vi "TLB Native Dynamic Events ver 0.14a.vi"() -> ()   [LabVIEW 2018]
uses:
  Labview Training Phase 2/Enum Controls/States for Action Engine.ctl
  TLB Type Definitions/State Type Definitions, for 0.26d versions and later.ctl
  TLB Type Definitions/Intruction Type Definitions.ctl
  TLB Type Definitions/Encoder cluster.ctl
  TLB Type Definitions/PING CLUSTER.ctl
  <vilib>/Studica/Studica Toolkit/NavX/NavX.lvlib
  <vilib>/Studica/Studica Toolkit/Background/DIO Channel.ctl
  Underlying VI's/NavX VI/navX type def.ctl
  <vilib>/myRIO/Instrument Drivers/Utilities/Utilities.lvlib
  <vilib>/Studica/Studica Toolkit/Background/I2C Channel.ctl
  TLB Type Definitions/Vision cluster.ctl
  <vilib>/NI_Real-Time Target Support.lvlib
  TLB Type Definitions/Stepper cluster.ctl
  Experimental VI's/Archived VI's/MOTOR CONTROL NO PID Type Def.ctl
  Underlying VI's/I2C Master VI/I2C MASTER Type Def.ctl
  Underlying VI's/I2C Master VI/I2C_MASTER_WRITE_NEW Type Def.ctl
  <vilib>/userdefined/High Color/IMAQdx.ctl
  Underlying VI's/I2C Master VI/Arduino_Interfacing.ctl
  TLB Type Definitions/Yaw Cluster.ctl
  Experimental VI's/Archived VI's/MOTOR CONTROL NO PID AE DATA ENTRY MODE Type def.ctl
  Experimental VI's/Archived VI's/MOTOR CONTROL NO PID AE DIRECTIONS type def.ctl
  Underlying VI's/Elasped Timer/Control.ctl
  TLB Type Definitions/Time cluster.ctl
  TLB Type Definitions/Y Stepper cluster.ctl
  Underlying VI's/Modified webcam FGV/Webcam AE.ctl
  <vilib>/Utility/RT CPU Load.ctl
panel:
  out "Cluster":T1
  out "Object Center Coordinates":cluster{"x":sgl, "y":sgl}
  out "Object detection cluster":T2
  out "Time up flag":bool
  out "Speed & distance":T3
  out "Task selection":u8
  in  "Object recognition mode":enum16{"Ball", "Soap", "Gel", "Pipe", "None"}(ring)
  out "NavX Readings":T4
  out "Arduino Data":T5
  out "CPU loads":T6[](array[typedef]) {"ISR (%)" format="%#.2f"; "Idle (%)" format="%#.2f"; "Background (%)" format="%#.2f"; "Normal (%)" format="%#.2f"; "Above Normal (%)" format="%#.2f"; "High (%)" format="%#.2g"; "Timed Structures (%)" format="%#.2g"; "Time Critical (%)" format="%#.2g"; "Total (%)" format="%#.2g"}
  out "Obstacle detected?":bool
  out "TASK ENABLE":bool
  out "Rising Edge":bool
  in  "Green LED":bool
  out "Obstacle detected":bool
  out "I2C Error":errorcluster
  out "State Logic":T7=enum."Startup"
  out "elements":T8[](array[typedef])
  in  "STOP TASK":bool
  in  "OK Button":bool
  in  "STOP":bool
  out "error out":errorcluster
  out "Action Queue Items":i32
  out "State Logic Queue Items":i32
  out "Action Queues items":string[](array[string])=["Hardware reset", "Software reset", ""]
  out "Action State":string
  # "VISION"
  # "System Health Status Update"
  # "TLB FRAMEWORK STATUS"
  # "Test Programme written by Calvin Loke    Dated: 28 Aug 2019\nTest Programme revised by Dr Alex See   Dated 30 Aug 2019\n\nRevision date: 20/03/2020\nProgramme version:   TLB Native Dynamic Events ver 0.14a"
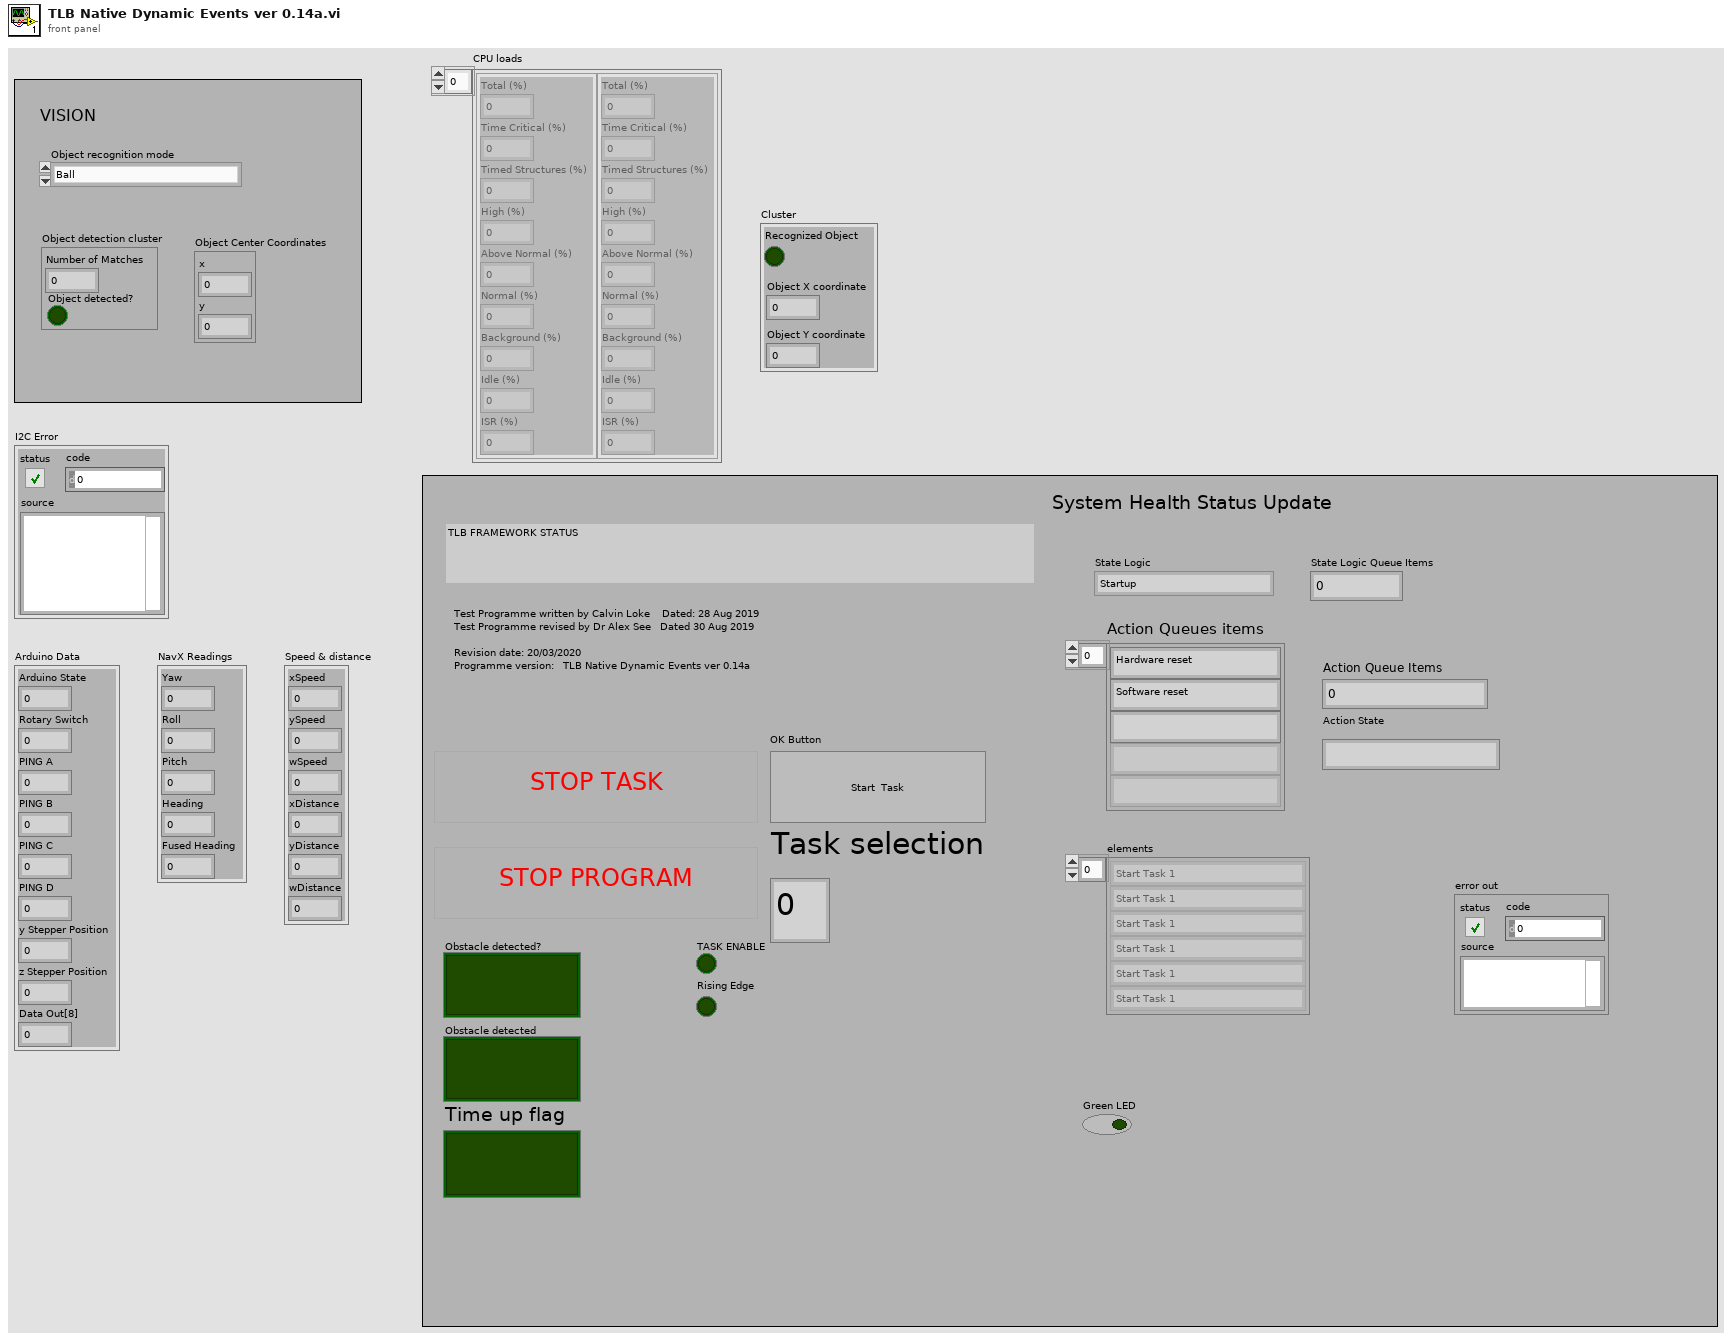
[diagram p1: front panel]
types:
  T1 = typedef "Vision cluster.ctl" = cluster{"Recognized Object":bool, "Object X coordinate":dbl, "Object Y coordinate":dbl}
  T2 = cluster{"Number of Matches":i32, "Object detected?":bool}
  T3 = cluster{"xSpeed":dbl, "ySpeed":dbl, "wSpeed":dbl, "xDistance":dbl, "yDistance":dbl, "wDistance":dbl}
  T4 = cluster{"Yaw":dbl, "Roll":dbl, "Pitch":dbl, "Heading":dbl, "Fused Heading":dbl}
  T5 = cluster{"Arduino State":u8, "Rotary Switch":u8, "PING A":u8, "PING B":u8, "PING C":u8, "PING D":u8, "y Stepper Position":u8, "z Stepper Position":u8, "Data Out[8]":u8}
  T6 = typedef "NI_Real-Time Target Support.lvlib/RT CPU Load.ctl" = cluster{"Total (%)":dbl, "Time Critical (%)":dbl, "Timed Structures (%)":dbl, "High (%)":dbl, "Above Normal (%)":dbl, "Normal (%)":dbl, "Background (%)":dbl, "Idle (%)":dbl, "ISR (%)":dbl}
  T7 = typedef "State Type Definitions.ctl" = enum16{"None", "Startup", "Move to Angle", "True Stop", "Idle", "Shutdown", "Task 1A", "Task 1B", "Task 2:Raise Arm", "Task 2:Sensor Mode", "Task 2:Reverse Mode", "Task 3", "Task 4_A", "Task 4_B", "Task 4_C", "Task 4_D", "Task 5A", "Task 5B", "Task 5C", "Task 5D", "Task 5E: POSITION ARM", "Task 5F: ARM GRAB HEIGHT", "Task 5G: CLOSE CLAW", "Task 5H: RAISE ARM", "Task 6_A", "Task 6_B", "Task 7", "Task 8A: RAISE ARM", "Task 8B: MOVE TO BOX", "Task 8C: CAM BURST", "Task 8D: PROCESS IMAGE", "Task 8E: ROBOT ADJUST", "Task 8F: CAM BURST 2", "Task 8G: PROCESS IMAGE 2", "Task 8H: ARM ADJUST", "Task 8I: ARM GRAB HEIGHT", "Task 8J: CLOSE CLAW", "Task 8K: RAISE MY SWORD", "Task 9A: Raise Arm", "Task 9B: Rotate to Angle", "Task 9C: Detect Box", "Task 9D: MOVE FORWARD", "Task 9E: MOVE LEFT", "Task 9F: SCAN IMAGE", "Task 9G: PROCESS COLOUR", "Task 9H: MOVE RIGHT", "Task 9I: SCAN IMAGE", "Task 9J: PROCESS COLOUR", "Task 9K: ROTATE 90 CW", "Task 9L: MOVE FORWARD", "Task 9M: MOVE RIGHT", "Task 9N: SCAN IMAGE", "Task 9O: PROCESS COLOUR", "Task 9P: MOVE RIGHT", "Task 9Q: SCAN IMAGE", "Task 9R: PROCESS COLOUR", "Task A1: Raise Arm", "Task A2: Rotate to Angle", "Task A3: Move Forward", "Task A4: Rotate CW 90"}
  T8 = typedef "Intruction Type Definitions.ctl" = enum16{"None", "Start Task 1", "Start Task 2", "Start Task 3", "Start Task 4", "Start Task 5", "Start Task 6", "Start Task 7", "Start Task 8 - BALL", "Start Task 8 - Gel", "Start Task 8 - Pipe", "Start Task 8 - Soap", "Start Task 9", "Start Task A", "Start Task B", "Exit"}
  T9 = typedef "Y Stepper cluster.ctl" = cluster{"yStepper desired":u8}
  T10 = typedef "Time cluster.ctl" = cluster{"Time up flag":bool, "SET TIME TO CHECK":dbl}
  T11 = typedef "Yaw Cluster.ctl" = cluster{"Yaw":dbl, "Compass":dbl}
  T12 = typedef "Stepper cluster.ctl" = cluster{"y Stepper Position":u8, "z Stepper Position":u8}
  T13 = typedef "DIO Channel.ctl" = enum16{"Not Connected", "A/DIO1", "A/DIO2", "A/DIO3", "A/DIO4", "A/DIO5", "A/DIO6", "A/DIO7", "A/DIO13", "B/DIO1", "B/DIO2", "B/DIO3", "B/DIO4", "B/DIO5", "B/DIO6", "B/DIO7", "B/DIO13", "C/DIO0", "C/DIO1", "C/DIO2", "C/DIO3", "C/DIO4", "C/DIO5", "C/DIO6", "C/DIO7"}
  T14 = typedef "PING CLUSTER.ctl" = cluster{"PING_A":u8, "PING_B":u8, "PING_C":u8, "PING_D":u8}
  T15 = typedef "Encoder cluster.ctl" = cluster{"xDistance":dbl, "yDistance":dbl, "wDistance":dbl}
  T16 = cluster{"DIO Channel":T13, "FPGA VI Reference Out":refnum<k20>}
  T17 = typedef "MOTOR CONTROL NO PID AE DATA ENTRY MODE Type def.ctl" = enum16{"Initialize", "Reset Encoders", "Write to motors", "Read from Encoders"}
  T18 = typedef "navX type def.ctl" = enum16{"Get i2C reference", "Read Values", "Zero Yaw"}
  T19 = typedef "Arduino_Interfacing.ctl" = enum16{"Initialize", "Write to Arduino", "Read From Arduino"}
  T20 = typedef "I2C Channel.ctl" = enum16{"Not Connected", "A", "B"}
  T21 = typedef "States for Action Engine.ctl" = enum16{"Initialize", "Write", "Read"}
  T22 = cluster{"I2C Ref Out":cluster{"I2C Channel":T20, "FPGA VI Reference Out":refnum<k20>}, "Connected":bool, "Slave Address (7-bit)":u8, "Registry":u8[]}
  T23 = typedef "IMAQ Image.ctl" = refnum<image>
  T24 = typedef "State Type Definitions.ctl" = enum16{"None", "Startup", "Move to Angle", "True Stop", "Idle", "Shutdown", "Task 1", "Task 2", "Task 3", "Task 4_A", "Task 4_B", "Task 4_C", "Task 4_D", "Task 5_A", "Task 5 _B", "Task 5_C", "Task 5_D", "Task 5_D_Error", "Task 5D_Error_Right", "Task 5D_Error_Left", "Task 5_E", "Task 5_F", "Task 5F_Error", "Task 5G", "Task 5H", "Task 6_A", "Task 6_B", "Task 7", "Task 8", "Task 9", "Task A", "Task B"}
  T25 = typedef "State Type Definitions.ctl" = enum16{"None", "Startup", "Move to Angle", "True Stop", "Idle", "Shutdown", "Task 1", "Task 2", "Task 3", "Task 4_A", "Task 4_B", "Task 4_C", "Task 5_A", "Task 5 _B", "Task 5_C", "Task 5_C_Error", "Task 5_D", "Task 6_A", "Task 6_B", "Task 7", "Task 8", "Task 9", "Task A", "Task B"}
  T26 = typedef "MOTOR CONTROL NO PID AE DIRECTIONS type def.ctl" = enum16{"y-axis movement", "x-axis movement", "Rotate", "Stop"}
  T27 = typedef "Control.ctl" = enum16{"Start", "Pause", "Initialize"}
  T28 = typedef "I2C_MASTER_WRITE_NEW Type Def.ctl" = enum16{"Ultrasonic sensors", "Stepper origin", "zStepper 13.3k", "zStepper 13k", "zStepper 12k", "zStepper 11k", "zStepper 10k", "zStepper 9k", "zStepper 8k", "zStepper 7k", "zStepper 6k", "zStepper 5k", "zStepper 4k", "zStepper 3k", "zStepper 2k", "zStepper 1k", "zStepper 900", "zStepper 800", "zStepper 700", "zStepper 600", "zStepper 500", "zStepper 400", "zStepper 300", "zStepper 200", "zStepper 100", "zStepper 0", "yStepper control", "Open Claw", "Close Claw", "Soft Reset"}
  T29 = typedef "Webcam AE.ctl" = enum16{"Initialize Camera", "Open Camera", "Continuous Acquisition", "Close Camera", "Retrieve Image", "Dispose Camera Image Buffer"}
  T30 = typedef "IMAQdx.ctl" = refnum<k21>
  T31 = typedef "Webcam AE.ctl" = enum16{"Initialize Camera", "Open Camera", "Continuous Acquisition", "Close Camera", "Retrieve Image", "Dispose Image Buffers"}
  T32 = typedef "MOTOR CONTROL NO PID Type Def.ctl" = enum16{"Init", "Front Back", "Left Right", "Rotate", "Stop", "Latch"}
  T33 = typedef "I2C MASTER Type Def.ctl" = enum16{"Last State", "Mode 0", "Mode 1", "Mode 2", "Mode 3", "Mode 4", "Mode 5", "Mode 6", "Mode 7", "Mode 8", "Mode 9", "Mode 10"}
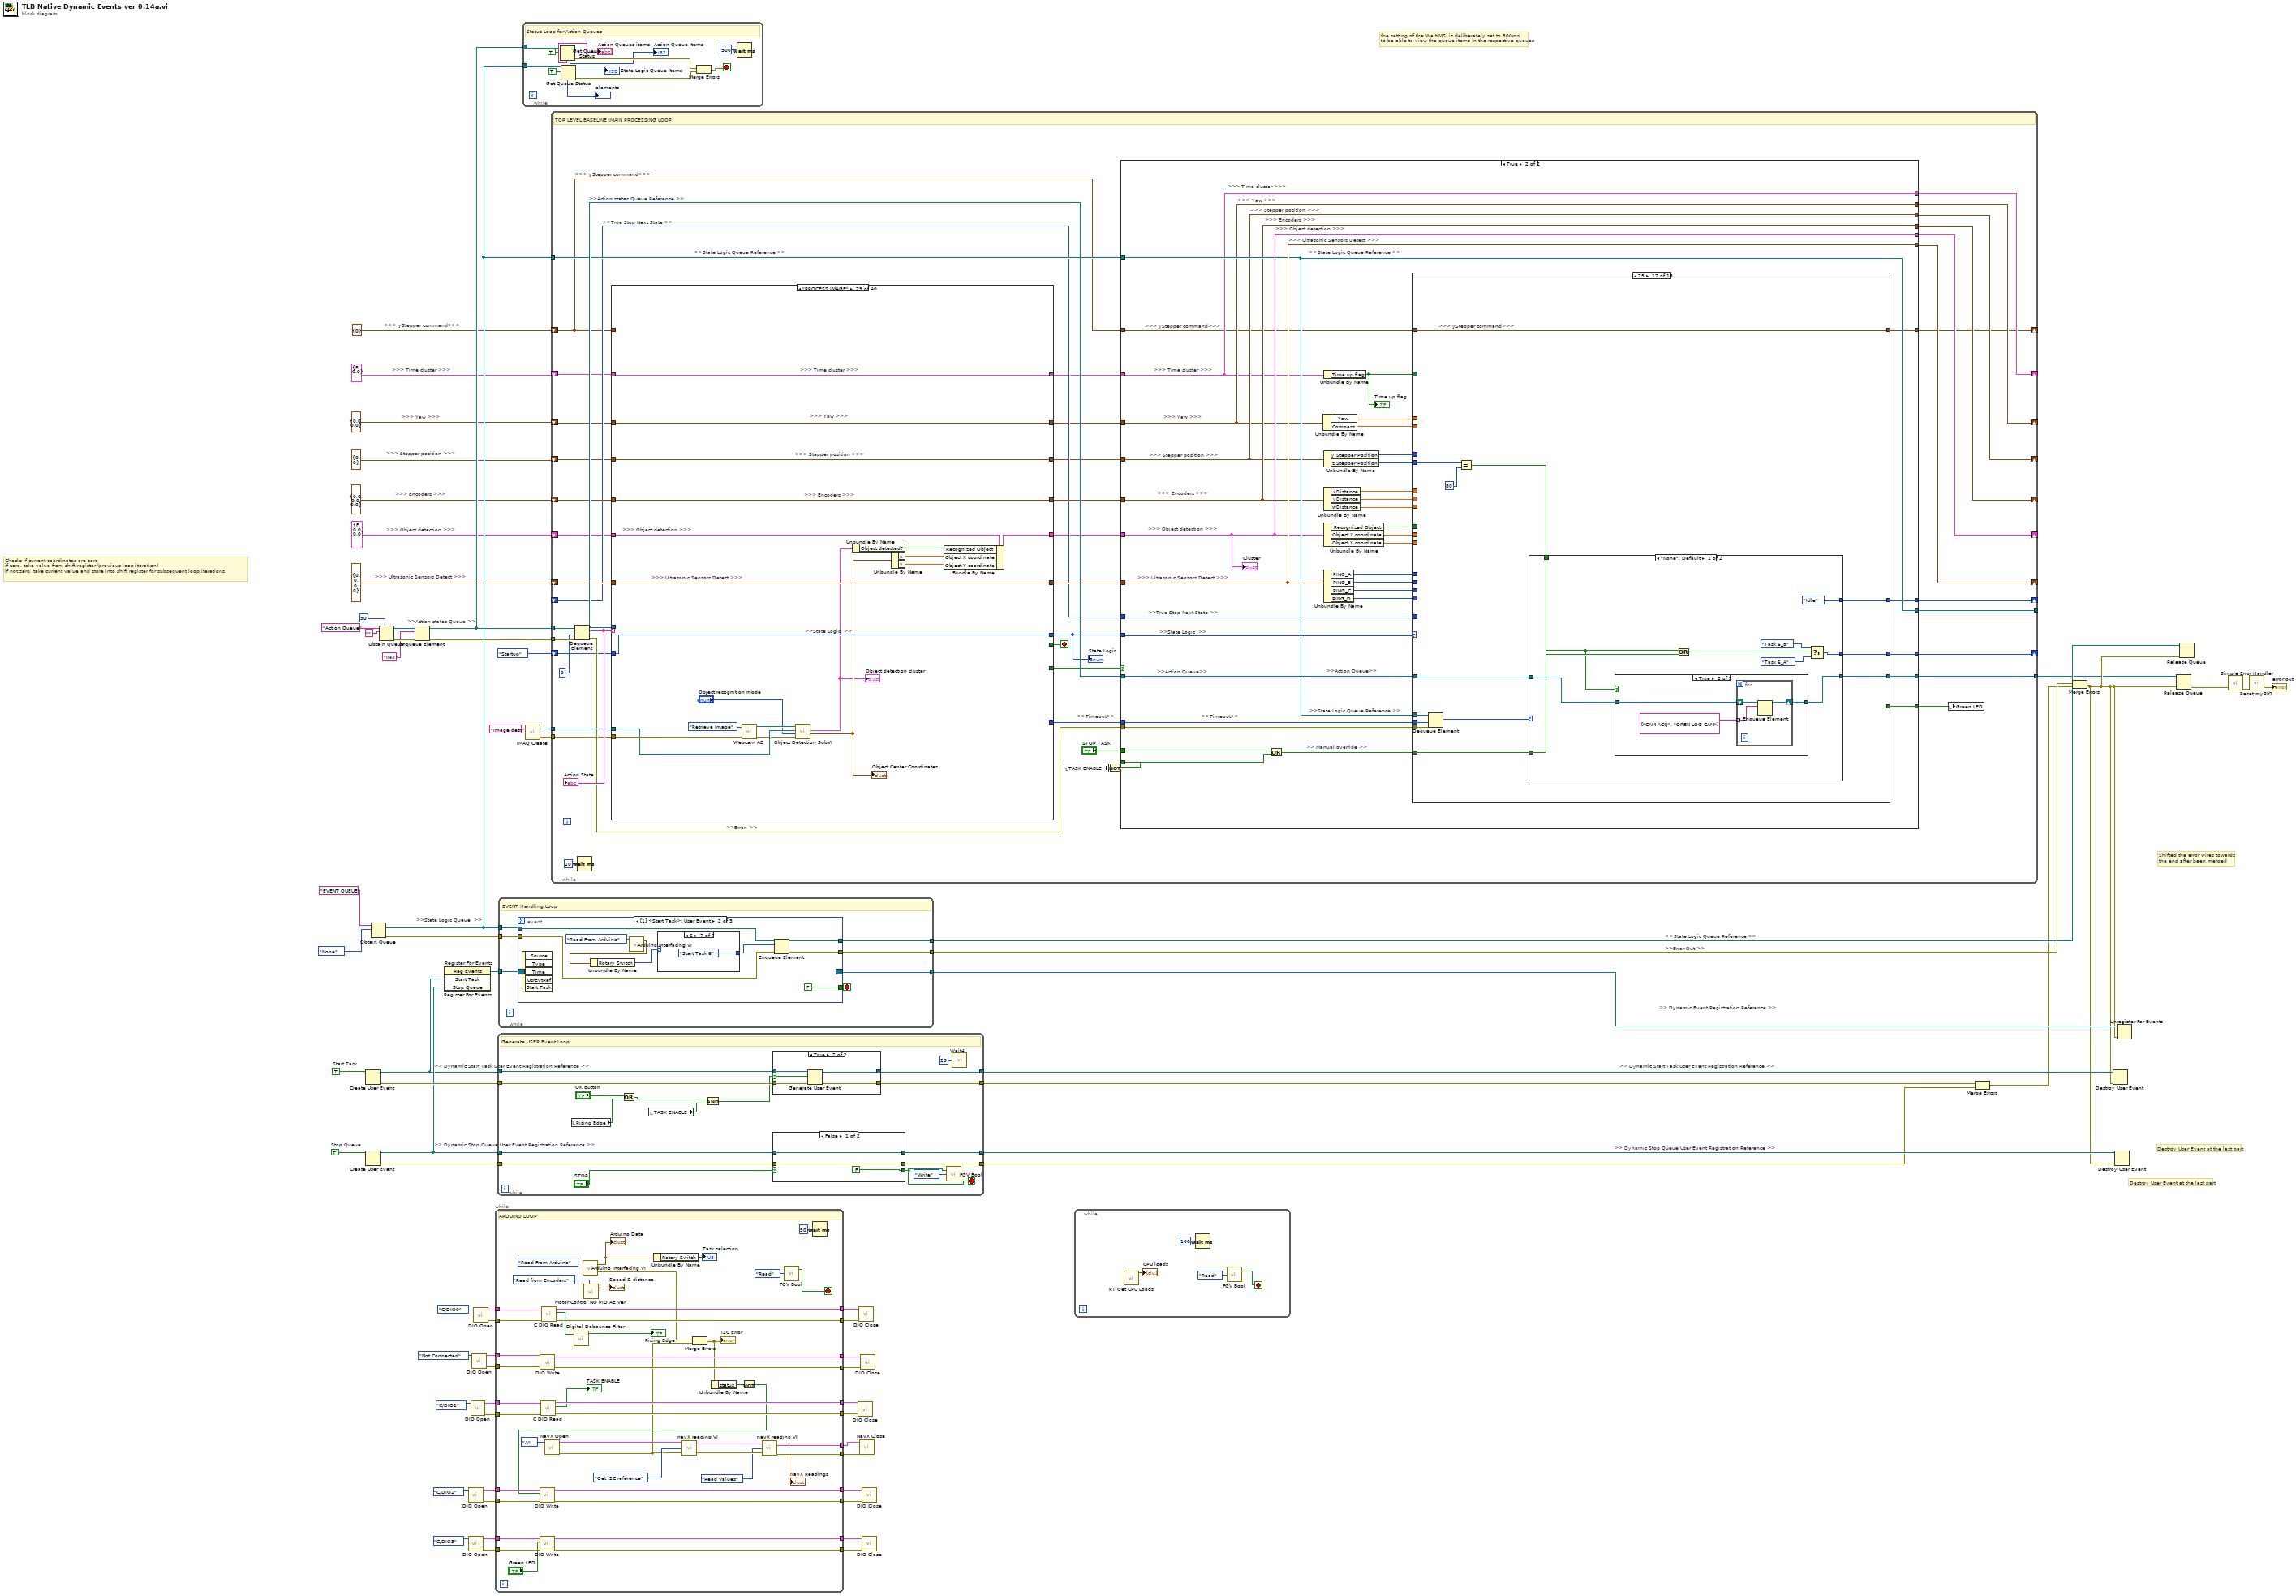
[diagram p0: block diagram]
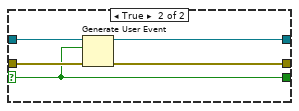
[diagram p2: hidden frame]
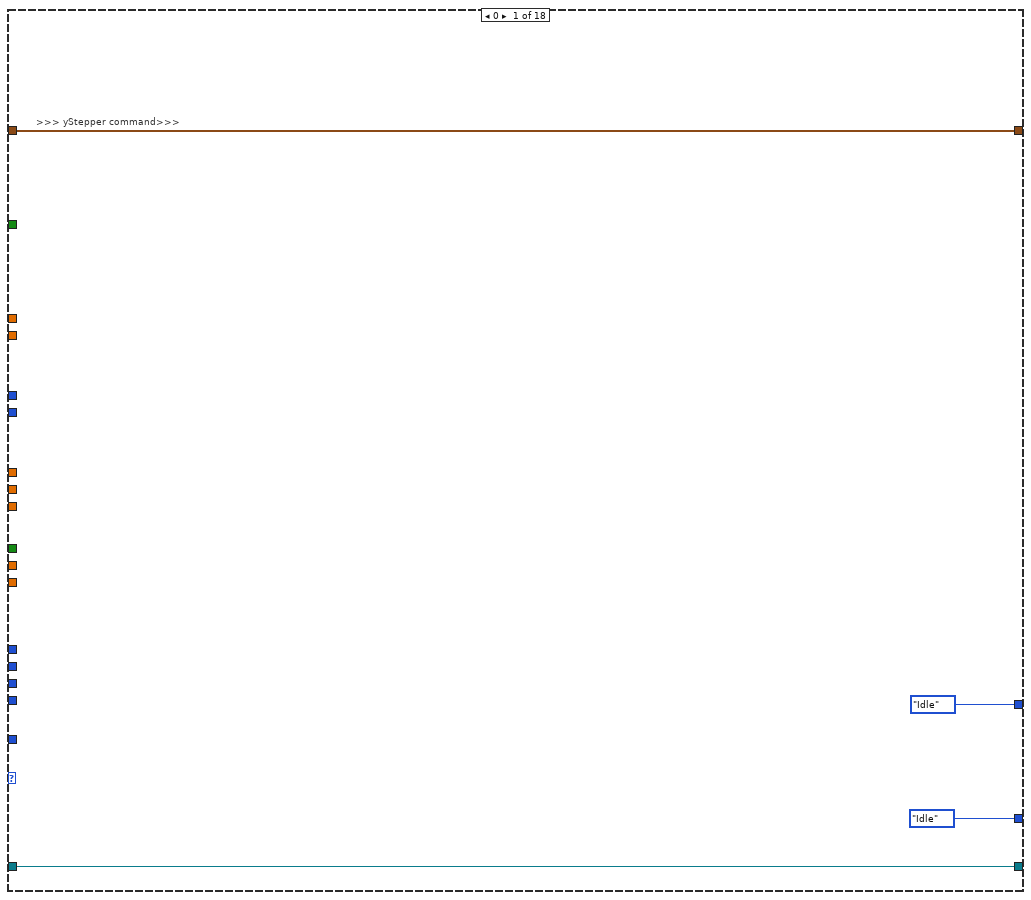
[diagram p5: hidden frame]
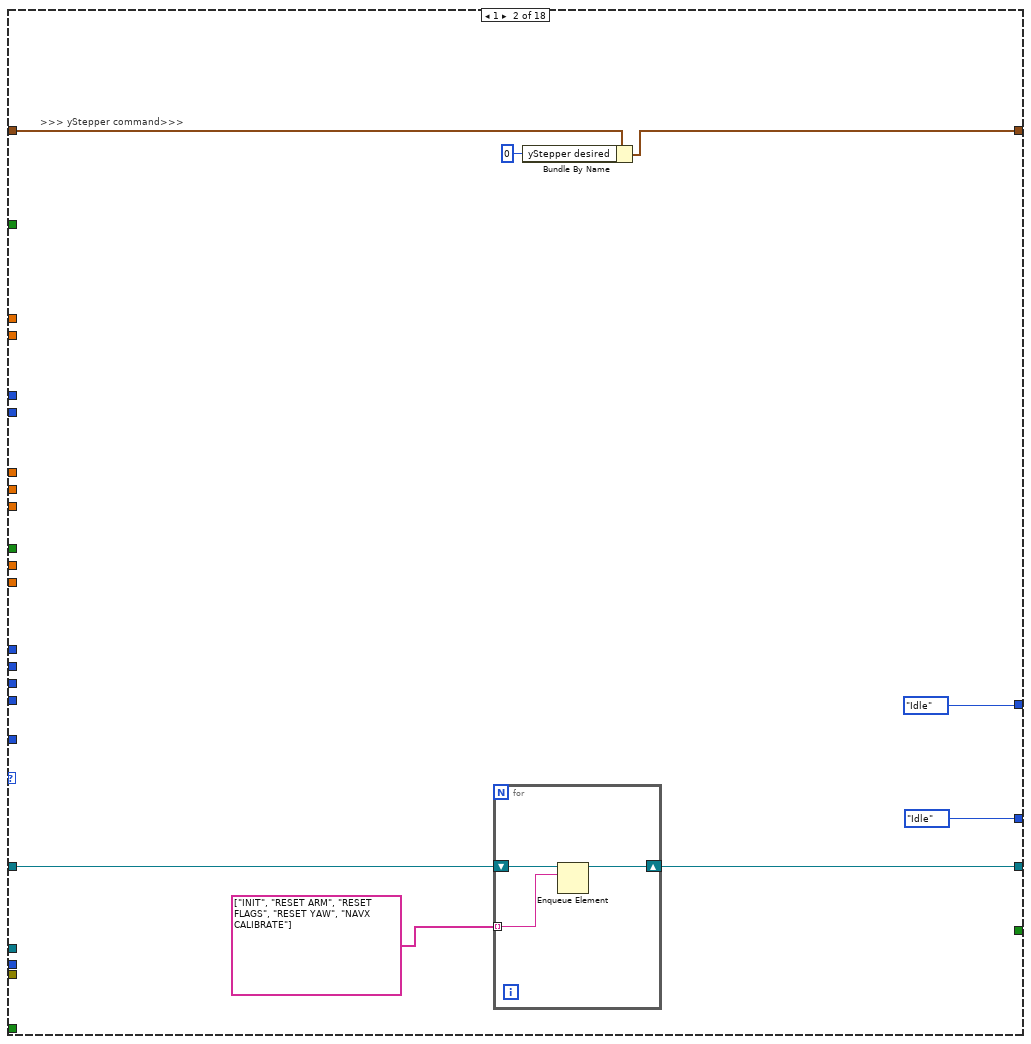
[diagram p6: hidden frame]
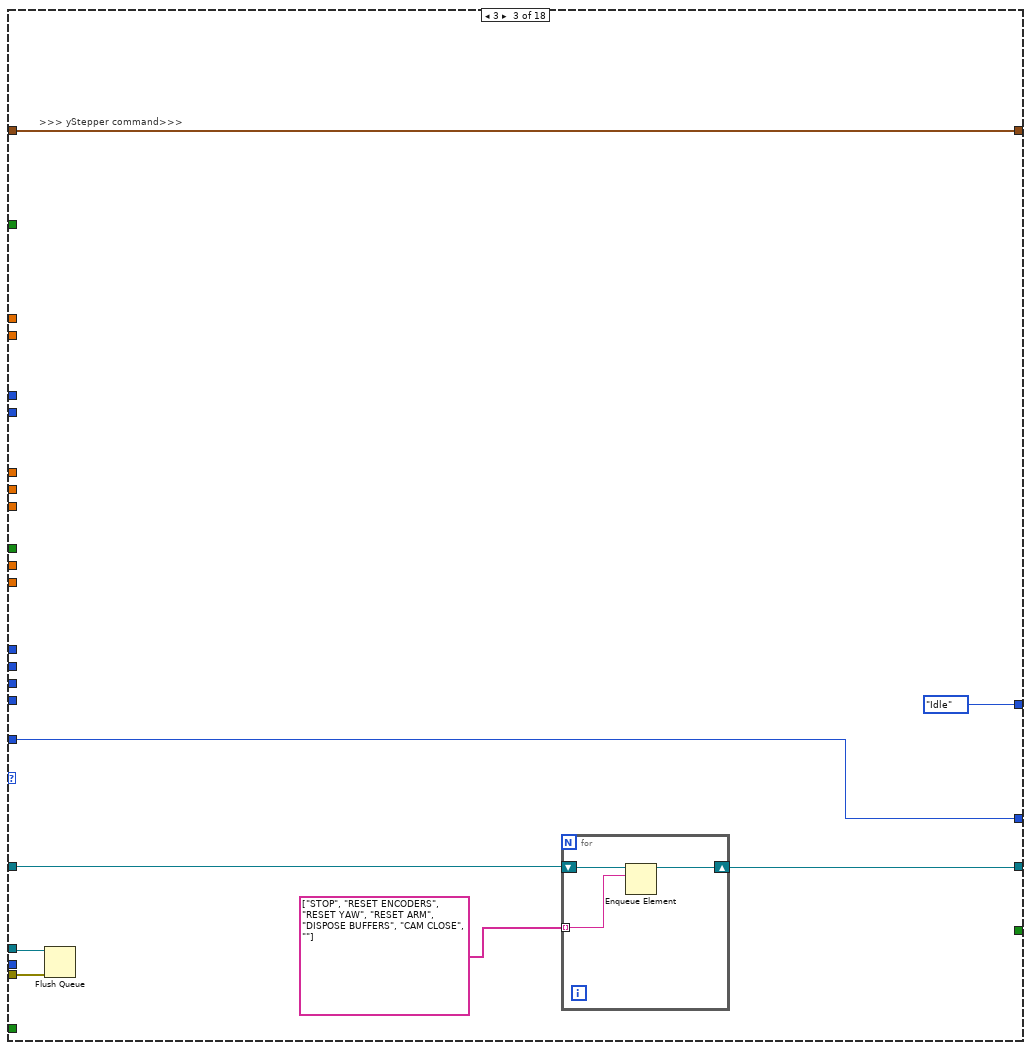
[diagram p7: hidden frame]
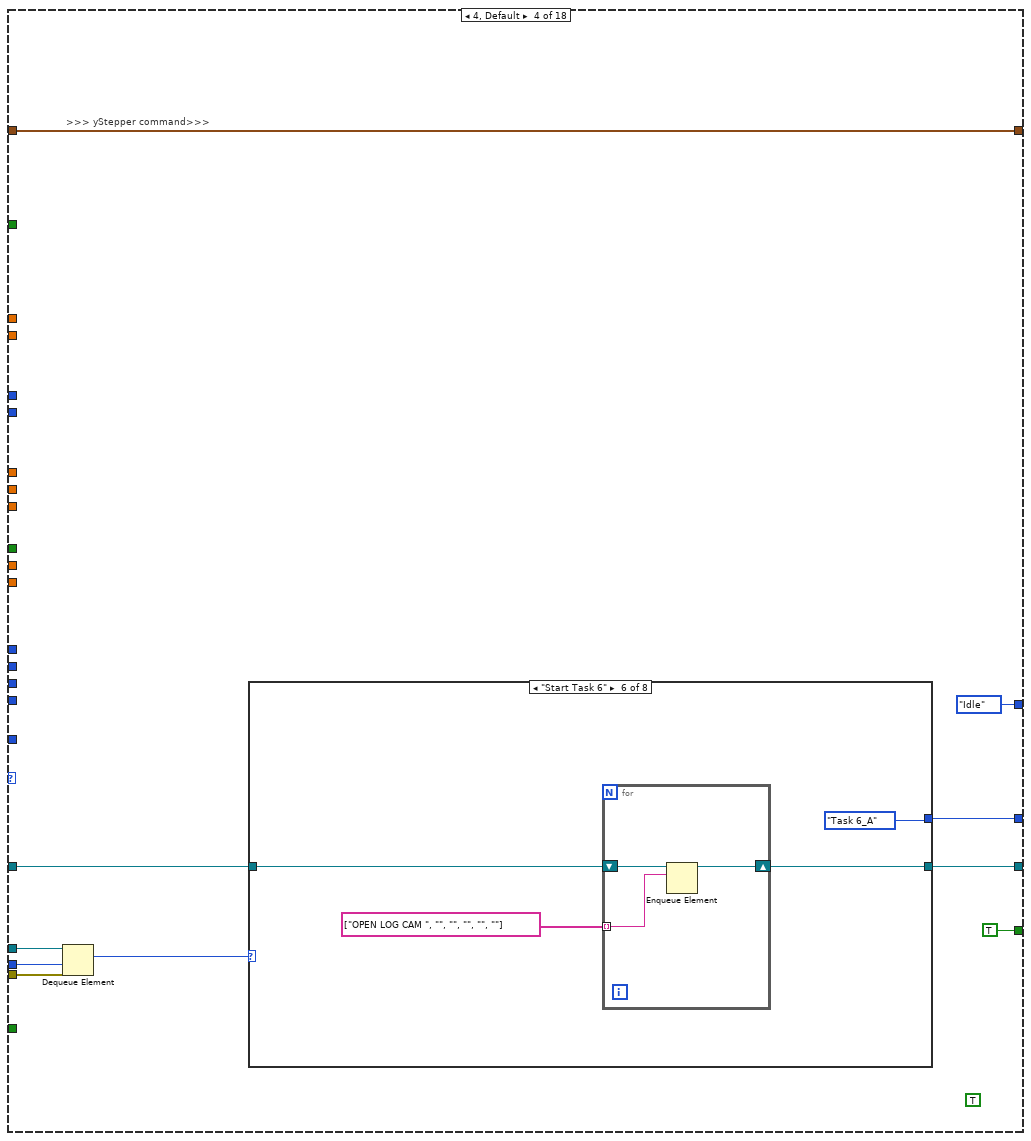
[diagram p8: hidden frame]
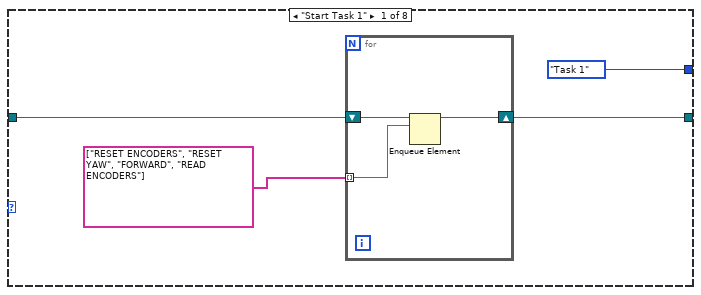
[diagram p9: hidden frame]
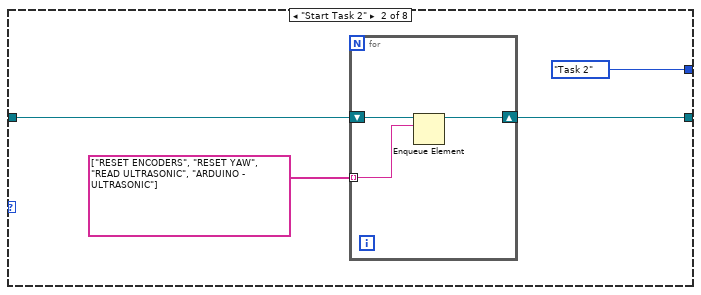
[diagram p10: hidden frame]
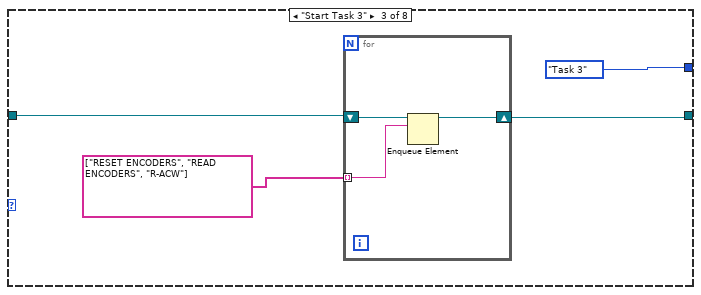
[diagram p11: hidden frame]
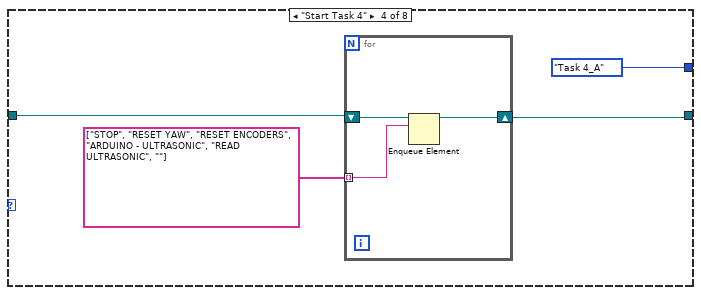
[diagram p12: hidden frame]
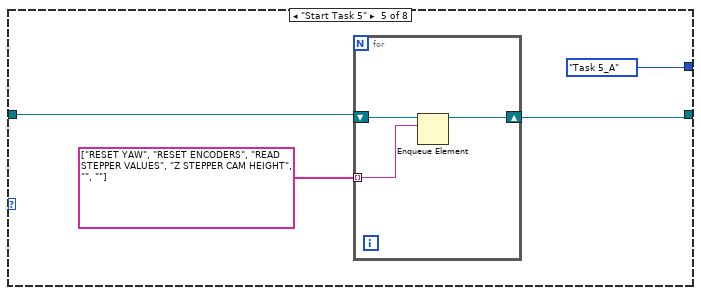
[diagram p13: hidden frame]
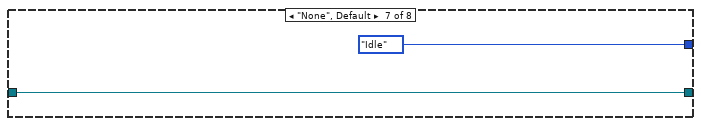
[diagram p14: hidden frame]
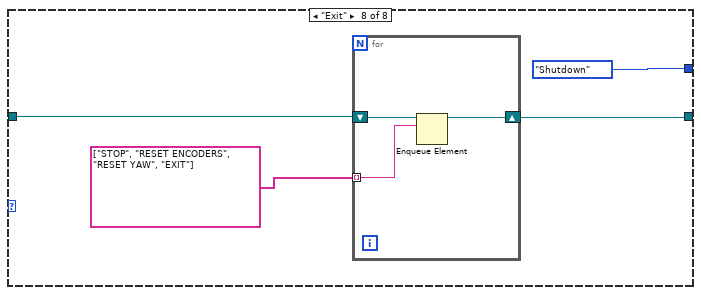
[diagram p15: hidden frame]
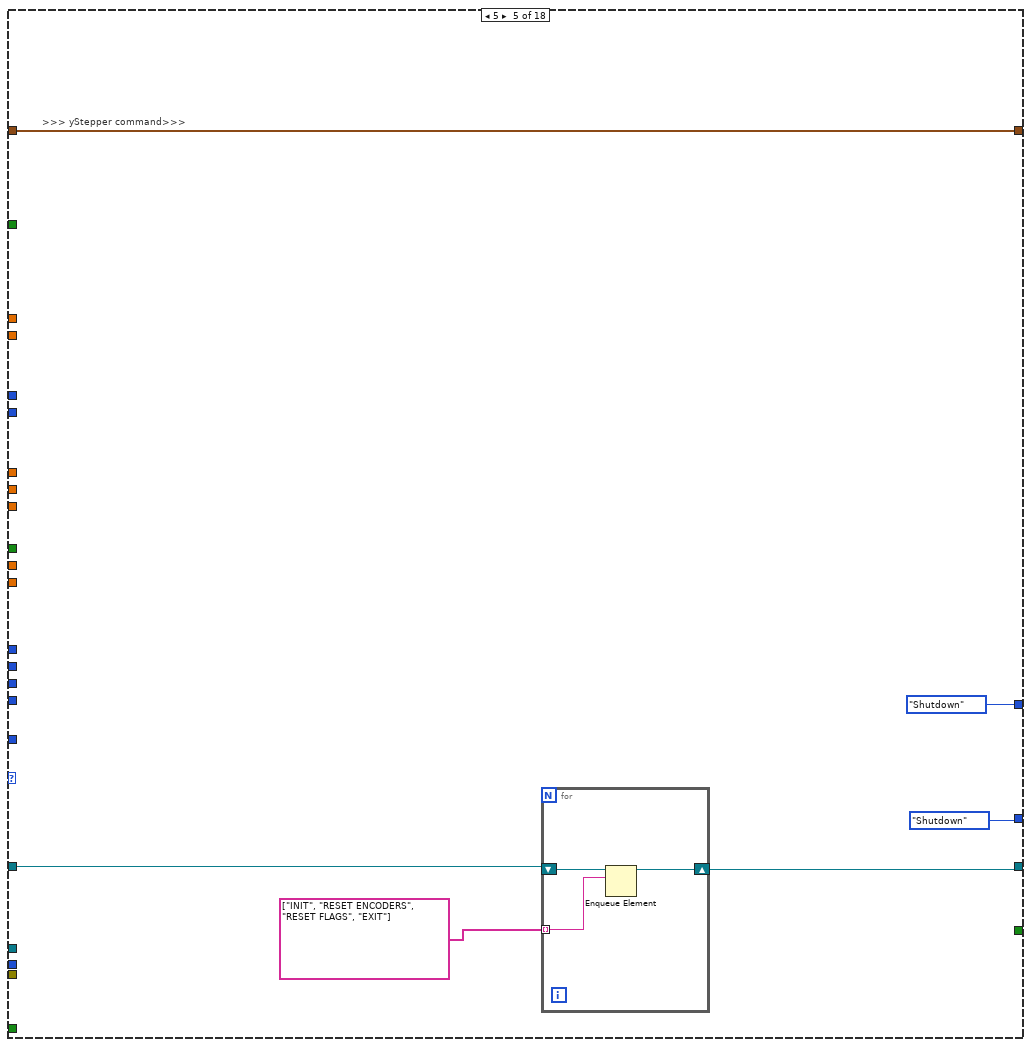
[diagram p16: hidden frame]
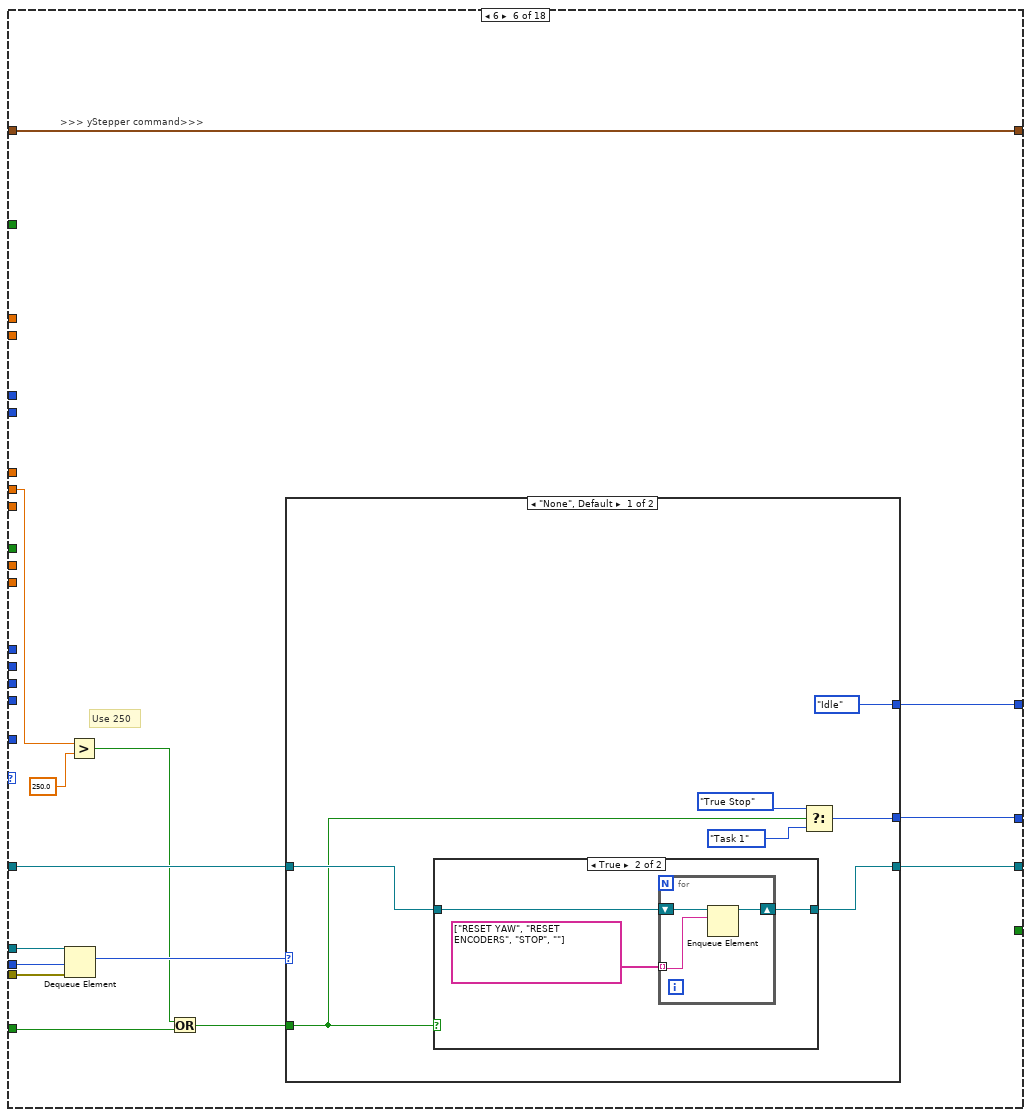
[diagram p17: hidden frame]
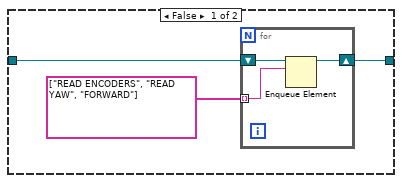
[diagram p18: hidden frame]
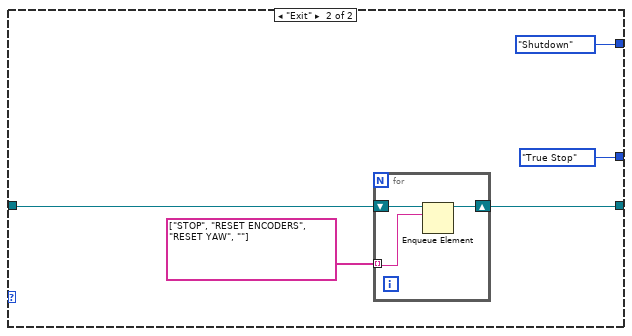
[diagram p19: hidden frame]
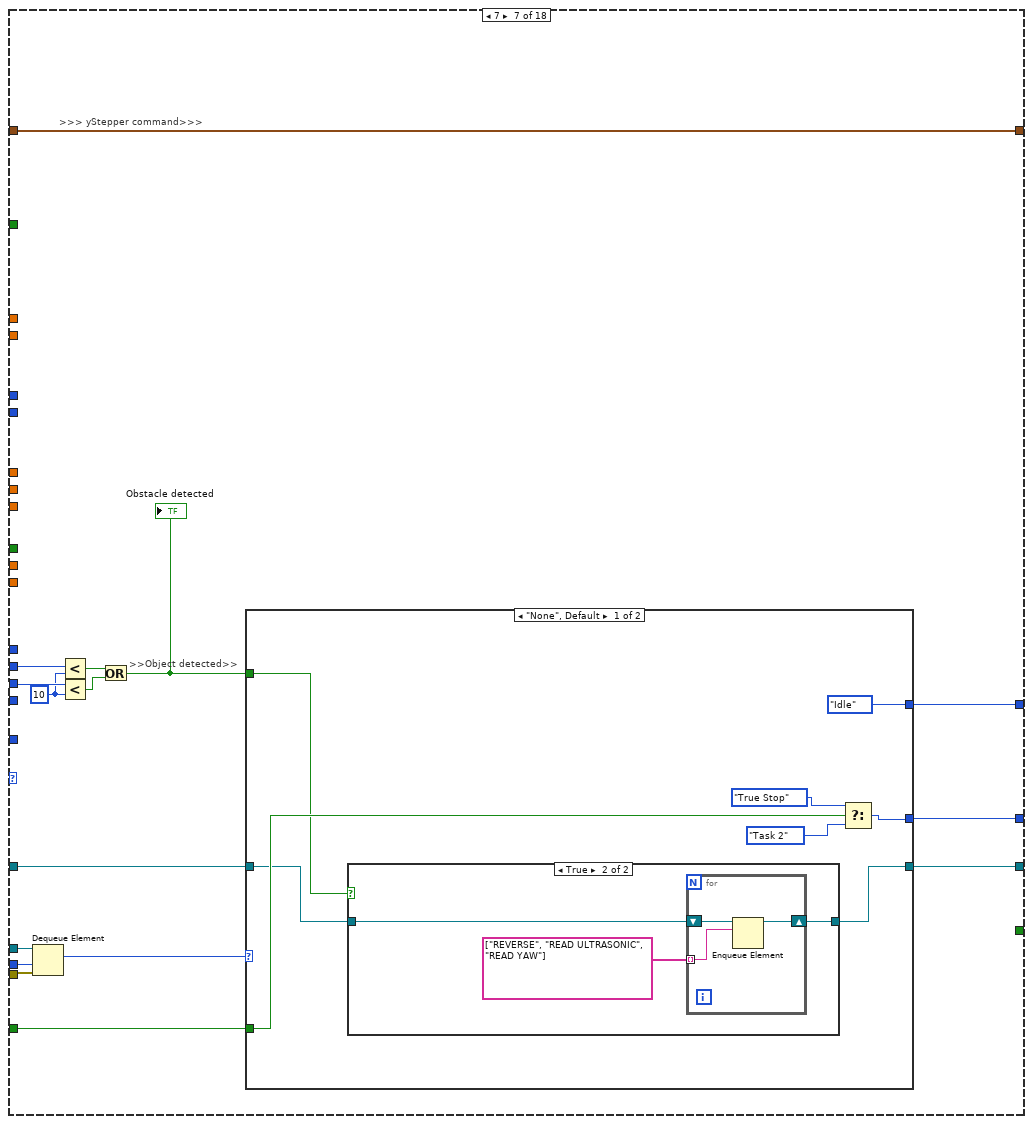
[diagram p20: hidden frame]
diagram:
  w70 = TRUE  # Stop Queue
  w69 = TRUE  # Start Task
  # "Checks if current coordinates are zero\nif zero, take value from shift register (previous loop iteration)\nif not zero, take current value and store into shift register for subsequent loop iterations"
  # ">>> yStepper command>>>"
  # ">>> Time cluster >>>"
  # ">>> Yaw >>>"
  # ">>> Stepper position >>>"
  # ">>> Encoders >>>"
  # ">>> Object detection >>>"
  # ">>> Ultrasonic Sensors Detect >>>"
  # "the setting of the Wait(MS) is deliberately set to 500ms\nto be able to view the queue items in the respective queues"
  # ">>Error Out >>"
  # ">> Dynamic Stop Queue User Event Registration Reference >>"
  # ">> Dynamic Start Task User Event Registration Reference >>"
  # ">> Dynamic Stop Queue User Event Registration Reference >>"
  # ">> Dynamic Start Task User Event Registration Reference >>"
  # ">> Dynamic Event Registration Reference >>"
  # ">>Action states Queue >>"
  # ">>State Logic Queue  >>"
  # ">>State Logic Queue Reference >>"
  # "Destroy User Event at the last part"
  # "Destroy User Event at the last part"
  # "Shifted the error wires towards\nthe end after been merged"
  n1 = Create User Event(user event datatype=w69) -> (user event=w61:refnum<user-event>, error out=w66:errorcluster)  [unwired: 1 in]
  n2 = Create User Event(user event datatype=w70) -> (user event=w62:refnum<user-event>, error out=w65:errorcluster)  [unwired: 1 in]
  n3 = Obtain Queue(name (unnamed)="EVENT QUEUE", element data type=Intruction_Type_Definitions."None" ("Enum")) -> (queue out=w47:refnum<queue>, error out=w53:errorcluster)  [unwired: 3 in, 1 out]
  n4 = Obtain Queue(max queue size (-1, unlimited)=50, name (unnamed)="Action Queue", element data type="") -> (queue out=w56:refnum<queue>, error out=w52:errorcluster)  [unwired: 2 in, 1 out]
  n5 = Enqueue Element(queue=w56, element="INIT", error in (no error)=w52) -> (queue out=w48:refnum<queue>, error out=w51:errorcluster)  [unwired: 1 in, 1 out]
  n6 = register-events "Register For Events"(w61, w62) -> (reference out=w60:refnum<event-registration>)  [unwired: 2 in, 1 out]
  n7 = call <vilib>:"DIO Open.vi"("DIO Channel"=DIO_Channel."C/DIO2") -> ("error out"=w14:errorcluster, "DIO Info Out"=w15:T16)  [unwired: 9 in]
  n8 = call <vilib>:"DIO Open.vi"("DIO Channel"=DIO_Channel."C/DIO3") -> ("error out"=w9:errorcluster, "DIO Info Out"=w10:T16)  [unwired: 9 in]
  n9 = call <vilib>:"DIO Open.vi"("DIO Channel"=DIO_Channel."C/DIO1") -> ("error out"=w25:errorcluster, "DIO Info Out"=w26:T16)  [unwired: 9 in]
  n10 = call <vilib>:"DIO Open.vi"("DIO Channel"=DIO_Channel."Not Connected") -> ("error out"=w30:errorcluster, "DIO Info Out"=w32:T16)  [unwired: 9 in]
  n11 = call <vilib>:"DIO Open.vi"("DIO Channel"=DIO_Channel."C/DIO0") -> ("error out"=w35:errorcluster, "DIO Info Out"=w38:T16)  [unwired: 9 in]
  n12 = while {
    tunnel: w38 -> [w113]
    tunnel: [w112] -> w36
    tunnel: w35 -> [w111]
    tunnel: [w110] -> w34
    tunnel: w32 -> [w107]
    tunnel: [w106] -> w31
    tunnel: w30 -> [w105]
    tunnel: [w104] -> w29
    tunnel: [w103] -> w27
    tunnel: w26 -> [w102]
    tunnel: w25 -> [w101]
    tunnel: [w100] -> w24
    tunnel: w15 -> [w94]
    tunnel: w14 -> [w93]
    tunnel: [w92] -> w13
    tunnel: [w91] -> w12
    tunnel: w10 -> [w90]
    tunnel: w9 -> [w89]
    tunnel: [w88] -> w8
    tunnel: [w87] -> w7
    tunnel: [w81] -> w4
    tunnel: [w80] -> w5
    stop <- w115 stop-if-true
    # "ARDUINO LOOP"
    n13 = call <vilib>:"DIO Write.vi"("error in (no error)"=w89, "Input"="Green LED", "DIO Info In"=w90) -> ("error out"=w87:errorcluster, "DIO Info Out"=w88:T16)  [unwired: 7 in]
    n14 = call <vilib>:"DIO Write.vi"("error in (no error)"=w105, "DIO Info In"=w107) -> ("error out"=w104:errorcluster, "DIO Info Out"=w106:T16)  [unwired: 8 in]
    n15 = call <vilib>:"C DIO Read.vi"("error in (no error)"=w101, "DIO Info In in"=w102) -> ("error out"=w100:errorcluster, "IN"=→"TASK ENABLE":bool, "DIO Info In out"=w103:T16)  [unwired: 7 in]
    n16 = call <vilib>:"C DIO Read.vi"("error in (no error)"=w111, "DIO Info In in"=w113) -> ("error out"=w110:errorcluster, "IN"=w109:bool, "DIO Info In out"=w112:T16)  [unwired: 7 in]
    n17 = call <vilib>:"NavX Open.vi"("I2C Channel"=I2C_Channel."A") -> ("error out"=w96:errorcluster, "NavX Info"=w98:T22)  [unwired: 9 in]
    n18 = call "Digital Debounce Filter.vi"("Boolean input"=w109) -> ("Rising Edge"=→"Rising Edge":bool)  [unwired: 1 in, 2 out]
    n19 = call "Arduino Interfacing VI.vi"("AE Mode"=Arduino_Interfacing."Read From Arduino") -> ("error out"=w84:errorcluster, "Arduino Data"=w77:T5)  [unwired: 3 in]
    "Arduino Data" <- w77
    n20 = call "Motor Control NO PID AE Ver.vi"("AE Mode"=MOTOR_CONTROL_NO_PID_AE_DATA_ENTRY_MODE_Type_def."Read from Encoders") -> ("Speed & distance"=→"Speed & distance":T3)  [unwired: 4 in, 1 out]
    n21 = Unbundle By Name(w77) -> ("Rotary Switch"=→"Task selection":u8)
    n22 = call "navX reading VI.vi"("NavX Info In"=w98, "Mode"=navX_type_def."Get i2C reference", "error in (no error)"=w96) -> ("NavX Info Out"=w83:T22, "Error Out"=w82:errorcluster)  [unwired: 2 out]
    n23 = Merge Errors(w84, w96) -> (w73:errorcluster)
    "I2C Error" <- w73
    n24 = Unbundle By Name(w73) -> ("status"=w72:bool)
    n25 = Not(x=w72) -> (.not. x?=w71:bool)
    n26 = call <vilib>:"DIO Write.vi"("error in (no error)"=w93, "Input"=w71, "DIO Info In"=w94) -> ("error out"=w91:errorcluster, "DIO Info Out"=w92:T16)  [unwired: 7 in]
    n27 = call "navX reading VI.vi"("NavX Info In"=w83, "Mode"=navX_type_def."Read Values", "error in (no error)"=w82) -> ("NavX Info Out"=w81:T22, "NavX Readings"=→"NavX Readings":T4, "Error Out"=w80:errorcluster)  [unwired: 1 out]
    n28 = call "FGV Bool.vi"("Init/Read/Write State"=States_for_Action_Engine."Read") -> ("Output node"=w115:bool)  [unwired: 2 in, 1 out]
    n29 = Wait (ms)(milliseconds to wait=u32 50) -> ()  [unwired: 1 out]
  }
  n30 = while {
    tunnel: w61 -> [w133]
    tunnel: w62 -> [w132]
    tunnel: [w131] -> w68
    tunnel: [w130] -> w67
    tunnel: w66 -> [w129]
    tunnel: [w128] -> w64
    tunnel: w65 -> [w127]
    tunnel: [w126] -> w63
    stop <- w124 stop-if-true
    # "Generate USER Event Loop"
    n31 = local read "Rising Edge"() -> (w120:bool)
    n32 = Or(x="OK Button", y=w120) -> (x .or. y?=w119:bool)
    n33 = local read "TASK ENABLE"() -> (w118:bool)
    n34 = And(x=w119, y=w118) -> (x .and. y?=w117:bool)
    n35 = case shown="True" w117 {
      selector: w117 -> [_ w144]
      tunnel: w133 -> [w143 w148]
      tunnel: [w143 w147] -> w130
      tunnel: w129 -> [w142 w146]
      tunnel: [w142 w145] -> w128
      frame False {
      }
      frame True {
        n36 = Generate User Event(user event=w148, event data cluster=w144, error in=w146) -> (user event out=w147:refnum<user-event>, error out=w145:errorcluster)  [unwired: 1 in]
      }
    }
    n37 = case shown="False" "STOP" {
      selector: "STOP" -> [_ w137]
      tunnel: w132 -> [w136 w141]
      tunnel: [w136 w140] -> w131
      tunnel: w127 -> [w135 w139]
      tunnel: [w135 w138] -> w126
      tunnel: [FALSE w137] -> w124
      frame False {
      }
      frame True {
        n38 = Generate User Event(user event=w141, event data cluster=w137, error in=w139) -> (user event out=w140:refnum<user-event>, error out=w138:errorcluster)  [unwired: 1 in]
      }
    }
    n39 = call "FGV Bool.vi"("Init/Read/Write State"=States_for_Action_Engine."Write", "Input Node"=w124) -> ()  [unwired: 1 in, 2 out]
    n40 = call "Wait4"("Count(uSec)"=u32 20) -> ()  [unwired: 1 out]
  }
  n41 = while {
    tunnel: w60 -> [w155]
    tunnel: [w154] -> w59
    tunnel: w47 -> [w152]
    tunnel: [w151] -> w58
    tunnel: w53 -> [w150]
    tunnel: [w149] -> w50
    stop <- w153 stop-if-true
    # "EVENT Handling Loop"
    n42 = event shown="[1] <Start Task>: User Event" {
      selector: w155 -> [_ _ _]
      dyn-events: [_ _ _] -> w154
      timeout: _ -> [_ _ _]
      tunnel: [FALSE FALSE w183] -> w153
      tunnel: w152 -> [w160 w169 w181]
      tunnel: [w159 w168 w182] -> w151
      tunnel: w150 -> [w158 w167 w180]
      tunnel: [w157 w166 w179] -> w149
      event Timeout {
        n43 = event-data() -> ()  [unwired: 1 in, 3 out]
        n44 = Enqueue Element(queue=w160, element=Intruction_Type_Definitions."None" ("Enum"), error in (no error)=w158) -> (queue out=w159:refnum<queue>, error out=w157:errorcluster)  [unwired: 1 in, 1 out]
      }
      event User Event {
        n45 = event-data() -> ()  [unwired: 1 in, 5 out]
        n46 = call "Arduino Interfacing VI.vi"("AE Mode"=Arduino_Interfacing."Read From Arduino") -> ("Arduino Data"=w163:T5)  [unwired: 3 in, 1 out]
        n47 = Unbundle By Name(w163) -> ("Rotary Switch"=w162:u8)
        n48 = case shown="6" w162 {
          tunnel: [Intruction_Type_Definitions."None" ("Enum") Intruction_Type_Definitions."Start Task 1" ("Enum") Intruction_Type_Definitions."Start Task 2" ("Enum") Intruction_Type_Definitions."Start Task 3" ("Enum") Intruction_Type_Definitions."Start Task 4" ("Enum") Intruction_Type_Definitions."Start Task 5" ("Enum") Intruction_Type_Definitions."Start Task 6" ("Enum")] -> w165
          frame 0, Default {
          }
          frame 1 {
          }
          frame 2 {
          }
          frame 3 {
          }
          frame 4 {
          }
          frame 5 {
          }
          frame 6 {
          }
        }
        n49 = Enqueue Element(queue=w169, element=w165, error in (no error)=w167) -> (queue out=w168:refnum<queue>, error out=w166:errorcluster)  [unwired: 1 in, 1 out]
      }
      event User Event {
        n50 = event-data() -> ("Stop Queue"=w183:bool)  [unwired: 1 in, 4 out]
        n51 = Enqueue Element At Opposite End(queue=w181, element=Intruction_Type_Definitions."Exit" ("Enum"), error in (no error)=w180) -> (queue out=w182:refnum<queue>, error out=w179:errorcluster)  [unwired: 1 in, 1 out]
      }
    }
  }
  n52 = while {
    tunnel: w48 -> [w193]
    tunnel: w47 -> [w190]
    stop <- w187 stop-if-true
    # "Status Loop for Action Queues"
    n53 = Get Queue Status(queue=w193, return elements? (F)=TRUE) -> (error out=w189:errorcluster, # elements in queue=→"Action Queue Items":i32, elements=→"Action Queues items":string[])  [unwired: 1 in, 5 out]
    n54 = Get Queue Status(queue=w190, return elements? (F)=TRUE) -> (# pending remove=→"State Logic Queue Items":i32, error out=w188:errorcluster, elements=→"elements":T8[])  [unwired: 1 in, 5 out]
    n55 = Merge Errors(w189, w188) -> (w187:errorcluster)
    n56 = Wait (ms)(milliseconds to wait=u32 500) -> ()  [unwired: 1 out]
  }
  n57 = call "IMAQ Create"("Image Name"="Image dest") -> ("New Image"=w19:T23, "error out"=w18:errorcluster)  [unwired: 4 in]
  n58 = while {
    tunnel: w47 -> [w227]
    tunnel: w48 -> [w239]
    tunnel: w51 -> [w237]
    tunnel: [w236] -> _
    tunnel: [w235] -> w41
    shift-right: [w228] -> _
    shift-left: T14 {"PING_A"=0, "PING_B"=0, "PING_C"=0, "PING_D"=0} -> [w230]
    shift-right: [w221] -> _
    shift-left: State_Type_Definitions."Startup" ("Enum") -> [w224]
    shift-right: [w217] -> _
    shift-left: T15 {"xDistance"=0.0, "yDistance"=0.0, "wDistance"=0.0} -> [w219]
    shift-right: [w214] -> _
    shift-left: _ -> [w213]
    tunnel: w19 -> [w212]
    tunnel: w18 -> [w211]
    shift-right: [w208] -> _
    shift-left: T1 {"Recognized Object"=FALSE, "Object X coordinate"=0.0, "Object Y coordinate"=0.0} -> [w210]
    shift-right: [w205] -> _
    shift-left: T12 {"y Stepper Position"=0, "z Stepper Position"=0} -> [w207]
    shift-right: [w202] -> _
    shift-left: T11 {"Yaw"=0.0, "Compass"=0.0} -> [w204]
    shift-right: [w199] -> _
    shift-left: T10 {"Time up flag"=FALSE, "SET TIME TO CHECK"=0.0} -> [w201]
    shift-right: [w197] -> _
    shift-left: T9 {"yStepper desired"=0} -> [w198]
    stop <- w226 stop-if-true
    # ">>> yStepper command>>>"
    # ">>True Stop Next State >>"
    # ">>Error  >>"
    # ">>Timeout>>"
    # ">>Action states Queue Reference >>"
    # ">>State Logic Queue Reference >>"
    # "TOP LEVEL BASELINE (MAIN PROCESSING LOOP)"
    n59 = Dequeue Element(queue=w239, timeout in ms (-1)=0, error in (no error)=w237) -> (queue out=w231:refnum<queue>, element=w238:string, error out=w232:errorcluster)  [unwired: 1 out]
    "Action State" <- w238
    n60 = Wait (ms)(milliseconds to wait=u32 20) -> ()  [unwired: 1 out]
    n61 = case shown="\"PROCESS IMAGE\"" w238 {
      tunnel: [_ _ _ _ _ _ _ _ _ _ _ _ _ _ _ _ 0 w1146 _ _ _ _ _ _ _ _ _ _ _ _ _ _ _ _ _ _ _ _ _ _] -> w234
      tunnel: w231 -> [_ _ _ _ _ _ _ _ _ _ _ _ _ _ _ _ _ _ _ _ _ _ _ _ _ _ _ _ _ _ _ _ _ _ _ _ _ _ _ _]
      tunnel: w230 -> [w961 w969 w980 w991 w1001 w1011 w1022 w1033 w1043 w1049 w1063 w1076 w1087 w1095 w1119 w1128 w1138 w1147 w1155 w1163 w1192 w1202 w1209 w1217 w1229 w1241 w1250 w1258 w1274 w1282 w1292 w1301 w1310 w1319 w1325 w1336 w1351 w1356 w1367 w1377]
      tunnel: [w961 w969 w980 w991 w1001 w1011 w1022 w1033 w1043 w1049 w1063 w1077 w1087 w1095 w1120 w1128 w1138 w1147 w1155 w1163 w1191 w1202 w1209 w1217 w1229 w1241 w1250 w1258 w1274 w1282 w1292 w1301 w1310 w1319 w1325 w1336 w1351 w1356 w1367 w1377] -> w229
      tunnel: [TRUE TRUE _ _ _ _ _ _ _ _ _ _ _ _ _ _ _ _ _ _ _ _ _ _ _ _ _ _ _ _ _ _ _ _ _ _ _ _ _ _] -> w226
      tunnel: w224 -> [w959 w967 w979 w990 w1000 w1010 w1021 w1032 w1042 w1048 w1062 w1075 w1086 w1094 w1118 w1127 w1135 w1144 w1154 w1162 w1190 w1201 w1208 w1216 w1228 w1240 w1249 w1257 w1273 w1281 w1291 w1300 w1309 w1318 w1324 w1335 w1350 w1355 w1366 w1376]
      tunnel: [_ _ _ _ _ _ _ _ _ _ _ _ _ _ _ _ _ TRUE _ _ _ _ _ _ _ _ _ _ _ _ _ _ _ _ _ _ _ _ _ _] -> w223
      tunnel: [w959 w967 w979 w990 w1000 w1010 w1021 w1032 w1042 w1048 w1062 w1075 w1086 w1094 w1118 w1127 w1135 w1144 w1154 w1162 w1190 w1201 w1208 w1216 w1228 w1240 w1249 w1257 w1273 w1281 w1291 w1300 w1309 w1318 w1324 w1335 w1350 w1355 w1366 w1376] -> w222
      tunnel: w219 -> [w958 w966 w978 w989 w999 w1009 w1020 w1031 w1041 w1050 w1061 w1074 w1088 w1096 w1117 w1129 w1134 w1143 w1156 w1164 w1180 w1200 w1211 w1218 w1230 w1242 w1251 w1259 w1275 w1284 w1294 w1303 w1312 w1321 w1327 w1338 w1353 w1358 w1369 w1379]
      tunnel: [w958 w966 w978 w989 w999 w1009 w1020 w1031 w1041 w1050 w1060 w1074 w1088 w1096 w1116 w1129 w1134 w1143 w1156 w1164 w1179 w1200 w1211 w1218 w1230 w1242 w1251 w1259 w1275 w1284 w1294 w1303 w1312 w1321 w1327 w1338 w1353 w1358 w1369 w1379] -> w218
      tunnel: w212 -> [w953 _ _ _ _ _ _ _ _ _ _ _ _ _ _ _ _ _ _ _ _ _ _ _ _ _ _ _ w1269 _ _ _ _ _ _ _ _ _ _ _]
      tunnel: w211 -> [_ _ _ _ _ _ _ _ _ _ _ _ _ _ _ _ _ _ _ _ _ _ _ _ _ _ w1243 _ w1271 w1280 _ _ _ _ _ _ _ _ _ _]
      tunnel: w210 -> [w957 w965 w977 w988 w998 w1008 w1019 w1030 w1039 w1047 w1059 w1073 w1081 w1093 w1108 w1126 w1133 w1142 w1153 w1161 w1185 w1198 w1210 w1215 w1227 w1239 w1245 w1256 w1266 w1283 w1293 w1302 w1311 w1320 w1326 w1337 w1352 w1357 w1368 w1378]
      tunnel: [w957 w965 w977 w988 w998 w1008 w1019 w1030 w1039 w1047 w1059 w1073 w1081 w1093 w1107 w1126 w1133 w1142 w1153 w1161 w1184 w1198 w1210 w1215 w1227 w1239 w1245 w1256 w1265 w1283 w1293 w1302 w1311 w1320 w1326 w1337 w1352 w1357 w1368 w1378] -> w209
      tunnel: w207 -> [w956 w964 w976 w987 w997 w1007 w1018 w1029 w1038 w1046 w1058 w1072 w1089 w1092 w1113 w1125 w1132 w1141 w1152 w1160 w1175 w1197 w1207 w1214 w1226 w1238 w1248 w1255 w1276 w1285 w1290 w1299 w1308 w1317 w1328 w1339 w1349 w1359 w1370 w1380]
      tunnel: [w956 w964 w976 w987 w997 w1007 w1018 w1029 w1038 w1046 w1058 w1072 w1089 w1092 w1112 w1125 w1132 w1141 w1152 w1160 w1174 w1197 w1207 w1214 w1226 w1238 w1248 w1255 w1276 w1285 w1290 w1299 w1308 w1317 w1328 w1339 w1348 w1359 w1370 w1380] -> w206
      tunnel: w204 -> [w955 w963 w971 w982 w992 w1006 w1013 w1024 w1037 w1045 w1052 w1065 w1084 w1091 w1103 w1124 w1131 w1140 w1151 w1159 w1171 w1196 w1204 w1213 w1225 w1237 w1247 w1254 w1277 w1286 w1289 w1296 w1305 w1314 w1329 w1340 w1343 w1360 w1371 w1381]
      tunnel: [w955 w963 w971 w982 w992 w1006 w1013 w1024 w1037 w1045 w1052 w1065 w1083 w1091 w1102 w1124 w1131 w1140 w1151 w1159 w1170 w1196 w1204 w1213 w1225 w1237 w1247 w1254 w1277 w1286 w1289 w1296 w1305 w1314 w1329 w1340 w1343 w1360 w1371 w1381] -> w203
      tunnel: w201 -> [w952 w962 w972 w983 w993 w1002 w1014 w1025 w1034 w1044 w1051 w1064 w1080 w1090 w1097 w1121 w1130 w1139 w1150 w1157 w1168 w1194 w1203 w1212 w1224 w1236 w1246 w1253 w1278 w1287 w1288 w1295 w1304 w1313 w1330 w1341 w1342 w1354 w1364 w1374]
      tunnel: [w952 w962 w972 w983 w993 w1002 w1014 w1025 w1034 w1044 w1051 w1064 w1080 w1090 w1097 w1121 w1130 w1139 w1150 w1157 w1167 w1194 w1203 w1212 w1224 w1236 w1246 w1253 w1278 w1287 w1288 w1295 w1304 w1313 w1330 w1341 w1342 w1354 w1362 w1373] -> w200
      tunnel: w198 -> [_ _ _ _ _ _ _ _ _ _ _ _ _ _ _ _ _ _ _ _ _ _ _ _ _ _ _ _ _ _ _ _ _ _ _ w1332 _ _ _ _]
      frame "Exit" {
        # ">>State Logic  >>"
        # ">>> Time cluster >>>"
        # ">>> Yaw >>>"
        # ">>> Stepper position >>>"
        # ">>> Encoders >>>"
        # ">>> Object detection >>>"
        # ">>> Ultrasonic Sensors Detect >>>"
        n62 = call "Imaq Dispose"("All Images? (No)"=TRUE, "Image"=w953) -> ()  [unwired: 4 in, 1 out]
      }
      frame "----Movement States----" {
        # ">>State Logic  >>"
        # ">>> Time cluster >>>"
        # ">>> Yaw >>>"
        # ">>> Stepper position >>>"
        # ">>> Encoders >>>"
        # ">>> Object detection >>>"
        # ">>> Ultrasonic Sensors Detect >>>"
      }
      frame "FORWARD" {
        # ">>> Time cluster >>>"
        # ">>> Yaw >>>"
        # ">>> Stepper position >>>"
        # ">>> Encoders >>>"
        # ">>> Object detection >>>"
        # ">>> Ultrasonic Sensors Detect >>>"
        n63 = Unbundle By Name(w971) -> ("Yaw"=w970:dbl)
        n64 = call "Motor Control NO PID AE Ver.vi"("Direction"=MOTOR_CONTROL_NO_PID_AE_DIRECTIONS_type_def."y-axis movement", "AE Mode"=MOTOR_CONTROL_NO_PID_AE_DATA_ENTRY_MODE_Type_def."Write to motors", "Speed"=0.5, "Yaw"=w970) -> ()  [unwired: 1 in, 2 out]
      }
      frame "LEFT" {
        # ">>State Logic  >>"
        # ">>> Time cluster >>>"
        # ">>> Yaw >>>"
        # ">>> Stepper position >>>"
        # ">>> Encoders >>>"
        # ">>> Object detection >>>"
        # ">>> Ultrasonic Sensors Detect >>>"
        n65 = Unbundle By Name(w982) -> ("Yaw"=w981:dbl)
        n66 = call "Motor Control NO PID AE Ver.vi"("Direction"=MOTOR_CONTROL_NO_PID_AE_DIRECTIONS_type_def."x-axis movement", "AE Mode"=MOTOR_CONTROL_NO_PID_AE_DATA_ENTRY_MODE_Type_def."Write to motors", "Speed"=-0.5, "Yaw"=w981) -> ()  [unwired: 1 in, 2 out]
      }
      frame "R-ACW" {
        n67 = call "Motor Control NO PID AE Ver.vi"("Direction"=MOTOR_CONTROL_NO_PID_AE_DIRECTIONS_type_def."Rotate", "AE Mode"=MOTOR_CONTROL_NO_PID_AE_DATA_ENTRY_MODE_Type_def."Write to motors", "Speed"=0.25) -> ()  [unwired: 2 in, 2 out]
      }
      frame "R-CW" {
        (unwired) -0.2 ("Speed")
        n68 = call "Motor Control NO PID AE Ver.vi"("Direction"=MOTOR_CONTROL_NO_PID_AE_DIRECTIONS_type_def."Rotate", "AE Mode"=MOTOR_CONTROL_NO_PID_AE_DATA_ENTRY_MODE_Type_def."Write to motors", "Speed"=-0.5) -> ()  [unwired: 2 in, 2 out]
      }
      frame "RIGHT" {
        n69 = Unbundle By Name(w1013) -> ("Yaw"=w1012:dbl)
        n70 = call "Motor Control NO PID AE Ver.vi"("Direction"=MOTOR_CONTROL_NO_PID_AE_DIRECTIONS_type_def."x-axis movement", "AE Mode"=MOTOR_CONTROL_NO_PID_AE_DATA_ENTRY_MODE_Type_def."Write to motors", "Speed"=0.5, "Yaw"=w1012) -> ()  [unwired: 1 in, 2 out]
      }
      frame "REVERSE" {
        n71 = Unbundle By Name(w1024) -> ("Yaw"=w1023:dbl)
        n72 = call "Motor Control NO PID AE Ver.vi"("Direction"=MOTOR_CONTROL_NO_PID_AE_DIRECTIONS_type_def."y-axis movement", "AE Mode"=MOTOR_CONTROL_NO_PID_AE_DATA_ENTRY_MODE_Type_def."Write to motors", "Speed"=-0.5, "Yaw"=w1023) -> ()  [unwired: 1 in, 2 out]
      }
      frame "STOP" {
        n73 = Wait (ms)(milliseconds to wait=u32 500) -> ()  [unwired: 1 out]
        n74 = call "Motor Control NO PID AE Ver.vi"("Direction"=MOTOR_CONTROL_NO_PID_AE_DIRECTIONS_type_def."Stop", "AE Mode"=MOTOR_CONTROL_NO_PID_AE_DATA_ENTRY_MODE_Type_def."Write to motors") -> ()  [unwired: 3 in, 2 out]
      }
      frame "----SENSOR READING---- " {
      }
      frame "READ ENCODERS" {
        # ">>> Time cluster >>>"
        # ">>> Yaw >>>"
        # ">>> Stepper position >>>"
        # ">>> Object detection >>>"
        # ">>> Current encoder distance >>>"
        # ">>> Ultrasonic Sensors Detect >>>"
        n75 = call "Motor Control NO PID AE Ver.vi"("AE Mode"=MOTOR_CONTROL_NO_PID_AE_DATA_ENTRY_MODE_Type_def."Read from Encoders") -> ("Speed & distance"=w1056:T3)  [unwired: 4 in, 1 out]
        n76 = Unbundle By Name(w1056) -> ("xDistance"=w1055:dbl, "yDistance"=w1054:dbl, "wDistance"=w1053:dbl)
        n77 = Bundle By Name(cluster=w1061, "xDistance"=w1055, "yDistance"=w1054, "wDistance"=w1053) -> (w1060:T15)
      }
      frame "READ ULTRASONIC" {
        (unwired) navX_type_def."Read Values" ("Mode")
        (unwired) MOTOR_CONTROL_NO_PID_Type_Def."Latch" ("Direction")
        # ">>> Ultrasonic Sensors Detect >>>"
        # ">>> Object detection >>>"
        # ">>> Encoders >>>"
        # ">>> Stepper position >>>"
        # ">>> Yaw >>>"
        n78 = call "Arduino Interfacing VI.vi"("AE Mode"=Arduino_Interfacing."Read From Arduino") -> ("Arduino Data"=w1070:T5)  [unwired: 3 in, 1 out]
        n79 = Unbundle By Name(w1070) -> ("PING A"=w1069:u8, "PING B"=w1068:u8, "PING C"=w1067:u8, "PING D"=w1066:u8)
        n80 = Bundle By Name(cluster=w1076, "PING_A"=w1069, "PING_B"=w1068, "PING_C"=w1067, "PING_D"=w1066) -> (w1077:T14)
      }
      frame "READ YAW" {
        # ">>> Time cluster >>>"
        # ">>> Yaw >>>"
        # ">>> Ultrasonic Sensors Detect >>>"
        # ">>> Object detection >>>"
        # ">>> Encoders >>>"
        # ">>> Stepper position >>>"
        n81 = call "navX reading VI.vi"("Mode"=navX_type_def."Read Values") -> ("NavX Readings"=w1079:T4)  [unwired: 2 in, 3 out]
        n82 = Unbundle By Name(w1079) -> ("Heading"=w1078:dbl)
        n83 = Unbundle By Name(w1079) -> ("Yaw"=w1082:dbl)
        n84 = Bundle By Name(cluster=w1084, "Yaw"=w1082, "Compass"=w1078) -> (w1083:T11)
      }
      frame "----SYSTEM MODES----" {
        (unwired) I2C_MASTER_Type_Def."Last State" ("Arduino Mode")
        # ">>> Object detection >>>"
        # ">>> Yaw >>>"
        # ">>> Ultrasonic Sensors Detect >>>"
        # ">>> Encoders >>>"
        # ">>> Stepper position >>>"
      }
      frame "INIT" {
        w1114 = u8 0
        w1115 = 0.0
        # ">>> Time cluster >>>"
        # ">>> Object detection >>>"
        # ">>> Yaw >>>"
        # ">>> Ultrasonic Sensors Detect >>>"
        # ">>> Encoders >>>"
        # ">>> Stepper position >>>"
        # ">>State Logic  >>"
        n85 = call "Arduino Interfacing VI.vi"("AE Mode"=Arduino_Interfacing."Initialize") -> ()  [unwired: 3 in, 2 out]
        n86 = call "FGV Bool.vi"("Init/Read/Write State"=States_for_Action_Engine."Initialize") -> ()  [unwired: 2 in, 2 out]
        n87 = call "Motor Control NO PID AE Ver.vi"("AE Mode"=MOTOR_CONTROL_NO_PID_AE_DATA_ENTRY_MODE_Type_def."Initialize") -> ()  [unwired: 4 in, 2 out]
        n88 = call "Elasped Timer.vi"("Action"=Control."Initialize") -> ()  [unwired: 7 in, 4 out]
        n89 = Bundle By Name(cluster=w1108, "Recognized Object"=FALSE, "Object X coordinate"=0.0, "Object Y coordinate"=0.0) -> (w1107:T1)
        n90 = Bundle By Name(cluster=w1113, "y Stepper Position"=u8 0, "z Stepper Position"=u8 0) -> (w1112:T12)
        n91 = Bundle By Name(cluster=w1117, "xDistance"=w1115, "yDistance"=w1115, "wDistance"=w1115) -> (w1116:T15)
        n92 = Bundle By Name(cluster=w1119, "PING_A"=w1114, "PING_B"=w1114, "PING_C"=w1114, "PING_D"=w1114) -> (w1120:T14)
        n93 = Bundle By Name(cluster=w1103, "Yaw"=0.0) -> (w1102:T11)
      }
      frame "ARDUINO - ULTRASONIC" {
        # ">>> Object detection >>>"
        # ">>> Yaw >>>"
        # ">>> Ultrasonic Sensors Detect >>>"
        # ">>> Encoders >>>"
        # ">>> Stepper position >>>"
        # ">>State Logic  >>"
        n94 = call "Arduino Interfacing VI.vi"("Data to Write"=I2C_MASTER_WRITE_NEW_Type_Def."Ultrasonic sensors", "AE Mode"=Arduino_Interfacing."Write to Arduino") -> ()  [unwired: 2 in, 2 out]
      }
      frame "NAVX CALIBRATE" {
        # ">>> Object detection >>>"
        # ">>> Yaw >>>"
        # ">>> Ultrasonic Sensors Detect >>>"
        # ">>> Encoders >>>"
        # ">>> Stepper position >>>"
        # ">>State Logic  >>"
        # "Adds a 15 second delay to the startup process \nfor the NavX to calibrate"
        n95 = Wait (ms)(milliseconds to wait=u32 5000) -> ()  [unwired: 1 out]
      }
      frame "NO ACTION", Default {
        (unwired) u8 0 ("y Stepper value")
        (unwired) TRUE ("Latch")
        (unwired) navX_type_def."Read Values" ("Mode")
        (unwired) MOTOR_CONTROL_NO_PID_Type_Def."Latch" ("Direction")
        # ">>> Object detection >>>"
        # ">>> Yaw >>>"
        # ">>> Ultrasonic Sensors Detect >>>"
        # ">>> Encoders >>>"
        # ">>> Stepper position >>>"
        # ">>State Logic  >>"
        n96 = case shown="4" w1144 {
          tunnel: [0 100] -> w1146
          frame 1, Default {
          }
          frame 4 {
          }
        }
      }
      frame "----RESET CASES----" {
        (unwired) I2C_MASTER_Type_Def."Last State" ("Arduino Mode")
        # ">>> Object detection >>>"
        # ">>> Yaw >>>"
        # ">>> Ultrasonic Sensors Detect >>>"
        # ">>> Encoders >>>"
        # ">>> Stepper position >>>"
        # ">>State Logic  >>"
      }
      frame "RESET ENCODERS" {
        # ">>> Object detection >>>"
        # ">>> Yaw >>>"
        # ">>> Ultrasonic Sensors Detect >>>"
        # ">>> Encoders >>>"
        # ">>> Stepper position >>>"
        # ">>State Logic  >>"
        n97 = call "Motor Control NO PID AE Ver.vi"("AE Mode"=MOTOR_CONTROL_NO_PID_AE_DATA_ENTRY_MODE_Type_def."Reset Encoders") -> ()  [unwired: 4 in, 2 out]
      }
      frame "RESET FLAGS" {
        (unwired) I2C_MASTER_Type_Def."Last State" ("Arduino Mode")
        # "Resets any software variables\nand/or non-critical states"
        n98 = Wait (ms)(milliseconds to wait=u32 20) -> ()  [unwired: 1 out]
        n99 = Bundle By Name(cluster=w1168, "Time up flag"=FALSE, "SET TIME TO CHECK"=0.0) -> (w1167:T10)
        n100 = Bundle By Name(cluster=w1185, "Recognized Object"=FALSE, "Object X coordinate"=0.0, "Object Y coordinate"=0.0) -> (w1184:T1)
        n101 = Bundle By Name(cluster=w1175, "y Stepper Position"=u8 0, "z Stepper Position"=u8 0) -> (w1174:T12)
        n102 = Bundle By Name(cluster=w1180, "xDistance"=0.0, "yDistance"=0.0, "wDistance"=0.0) -> (w1179:T15)
        n103 = Bundle By Name(cluster=w1192, "PING_A"=u8 0, "PING_B"=u8 0, "PING_C"=u8 0, "PING_D"=u8 0) -> (w1191:T14)
        n104 = Bundle By Name(cluster=w1171, "Yaw"=0.0) -> (w1170:T11)
      }
      frame "RESET YAW" {
        n105 = Wait (ms)(milliseconds to wait=u32 100) -> ()  [unwired: 1 out]
        n106 = call "navX reading VI.vi"("Mode"=navX_type_def."Zero Yaw") -> ()  [unwired: 2 in, 4 out]
      }
      frame "RESET ARM" {
        n107 = call "Arduino Interfacing VI.vi"("Data to Write"=I2C_MASTER_WRITE_NEW_Type_Def."Soft Reset", "AE Mode"=Arduino_Interfacing."Write to Arduino") -> ()  [unwired: 2 in, 2 out]
      }
      frame "--------CAM STATES-------" {
      }
      frame "OPEN LOG CAM" {
        n108 = call "Webcam AE.vi"("Session In"=T30 "cam0", "Camera states"=Webcam_AE."Initialize Camera") -> ("error out"=w1221:errorcluster, "Session Out"=w1220:T30)  [unwired: 1 in, 1 out]
        n109 = call "Webcam AE.vi"("error in (no error)"=w1221, "Session In"=w1220, "Camera states"=Webcam_AE."Open Camera") -> ()  [unwired: 3 out]
      }
      frame "OPEN LIFE CAM" {
        n110 = call "Webcam AE.vi"("Session In"=T30 "cam1", "Camera states"=Webcam_AE."Initialize Camera") -> ("error out"=w1233:errorcluster, "Session Out"=w1232:T30)  [unwired: 1 in, 1 out]
        n111 = call "Webcam AE.vi"("error in (no error)"=w1233, "Session In"=w1232, "Camera states"=Webcam_AE."Open Camera") -> ()  [unwired: 3 out]
      }
      frame "CAM ACQ" {
        # ">>State Logic  >>"
        # ">>> Time cluster >>>"
        # ">>> Yaw >>>"
        # ">>> Stepper position >>>"
        # ">>> Encoders >>>"
        # ">>> Object detection >>>"
        # ">>> Ultrasonic Sensors Detect >>>"
        n112 = call "Webcam AE.vi"("error in (no error)"=w1243, "Camera states"=Webcam_AE."Continuous Acquisition") -> ()  [unwired: 1 in, 3 out]
      }
      frame "CAM CLOSE" {
        # ">>State Logic  >>"
        # ">>> Time cluster >>>"
        # ">>> Yaw >>>"
        # ">>> Stepper position >>>"
        # ">>> Encoders >>>"
        # ">>> Object detection >>>"
        # ">>> Ultrasonic Sensors Detect >>>"
        n113 = call "Webcam AE.vi"("Camera states"=Webcam_AE."Close Camera") -> ()  [unwired: 2 in, 3 out]
      }
      frame "PROCESS IMAGE" {
        # ">>State Logic  >>"
        # ">>> Time cluster >>>"
        # ">>> Yaw >>>"
        # ">>> Stepper position >>>"
        # ">>> Encoders >>>"
        # ">>> Object detection >>>"
        # ">>> Ultrasonic Sensors Detect >>>"
        n114 = call "Webcam AE.vi"("error in (no error)"=w1271, "Camera states"=Webcam_AE."Retrieve Image") -> ("error out"=w1267:errorcluster, "Image Out"=w1270:T23)  [unwired: 1 in, 1 out]
        n115 = call "Object Detection SubVI.vi"("Error In"=w1267, "Mode"="Object recognition mode", "Image Dest"=w1269, "Image in"=w1270) -> ("Object Center Coordinates"=w1264:cluster{"x":sgl, "y":sgl}, "Object detection cluster"=w1260:T2)  [unwired: 2 out]
        "Object detection cluster" <- w1260
        "Object Center Coordinates" <- w1264
        n116 = Unbundle By Name(w1260) -> ("Object detected?"=w1261:bool)
        n117 = Unbundle By Name(w1264) -> ("x"=w1263:sgl, "y"=w1262:sgl)
        n118 = Bundle By Name(cluster=w1266, "Recognized Object"=w1261, "Object X coordinate"=w1263, "Object Y coordinate"=w1262) -> (w1265:T1)
      }
      frame "DISPOSE BUFFERS" {
        # ">>State Logic  >>"
        # ">>> Time cluster >>>"
        # ">>> Yaw >>>"
        # ">>> Stepper position >>>"
        # ">>> Encoders >>>"
        # ">>> Object detection >>>"
        # ">>> Ultrasonic Sensors Detect >>>"
        n119 = call "Webcam AE.vi"("error in (no error)"=w1280, "Camera states"=Webcam_AE."Dispose Image Buffers") -> ()  [unwired: 1 in, 3 out]
      }
      frame "-----ARM ACTIONS-----" {
      }
      frame "CLOSE CLAW" {
        n120 = call "Arduino Interfacing VI.vi"("Data to Write"=I2C_MASTER_WRITE_NEW_Type_Def."Close Claw", "AE Mode"=Arduino_Interfacing."Write to Arduino") -> ()  [unwired: 2 in, 2 out]
      }
      frame "OPEN CLAW" {
        n121 = call "Arduino Interfacing VI.vi"("Data to Write"=I2C_MASTER_WRITE_NEW_Type_Def."Open Claw", "AE Mode"=Arduino_Interfacing."Write to Arduino") -> ()  [unwired: 2 in, 2 out]
      }
      frame "Z STEPPER CAM HEIGHT" {
        n122 = call "Arduino Interfacing VI.vi"("Data to Write"=I2C_MASTER_WRITE_NEW_Type_Def."zStepper 8k", "AE Mode"=Arduino_Interfacing."Write to Arduino") -> ()  [unwired: 2 in, 2 out]
      }
      frame "Z STEPPER GRAB HEIGHT" {
        # ">>State Logic  >>"
        # ">>> Time cluster >>>"
        # ">>> Yaw >>>"
        # ">>> Stepper position >>>"
        # ">>> Encoders >>>"
        # ">>> Object detection >>>"
        # ">>> Ultrasonic Sensors Detect >>>"
        n123 = call "Arduino Interfacing VI.vi"("Data to Write"=I2C_MASTER_WRITE_NEW_Type_Def."zStepper 100", "AE Mode"=Arduino_Interfacing."Write to Arduino") -> ()  [unwired: 2 in, 2 out]
      }
      frame "Y STEPPER CONTROL" {
        # ">>State Logic  >>"
        # ">>> yStepper command>>>"
        # ">>> Time cluster >>>"
        # ">>> Yaw >>>"
        # ">>> Stepper position >>>"
        # ">>> Encoders >>>"
        # ">>> Object detection >>>"
        # ">>> Ultrasonic Sensors Detect >>>"
        n124 = Unbundle By Name(w1332) -> ("yStepper desired"=w1331:u8)
        n125 = call "Arduino Interfacing VI.vi"("y Stepper value"=w1331, "Data to Write"=I2C_MASTER_WRITE_NEW_Type_Def."yStepper control", "AE Mode"=Arduino_Interfacing."Write to Arduino") -> ()  [unwired: 1 in, 2 out]
      }
      frame "READ STEPPER VALUES" {
        # ">>State Logic  >>"
        # ">>> Time cluster >>>"
        # ">>> Yaw >>>"
        # ">>> Stepper position >>>"
        # ">>> Encoders >>>"
        # ">>> Object detection >>>"
        # ">>> Ultrasonic Sensors Detect >>>"
        n126 = call "Arduino Interfacing VI.vi"("AE Mode"=Arduino_Interfacing."Read From Arduino") -> ("Arduino Data"=w1346:T5)  [unwired: 3 in, 1 out]
        n127 = Unbundle By Name(w1346) -> ("y Stepper Position"=w1345:u8, "z Stepper Position"=w1344:u8)
        n128 = Bundle By Name(cluster=w1349, "y Stepper Position"=w1345, "z Stepper Position"=w1344) -> (w1348:T12)
      }
      frame " -----TIMING-----" {
        # ">>State Logic  >>"
        # ">>> Time cluster >>>"
        # ">>> Yaw >>>"
        # ">>> Stepper position >>>"
        # ">>> Encoders >>>"
        # ">>> Object detection >>>"
        # ">>> Ultrasonic Sensors Detect >>>"
      }
      frame "SET TIMER" {
        # ">>State Logic  >>"
        # ">>> Time cluster >>>"
        # ">>> Yaw >>>"
        # ">>> Stepper position >>>"
        # ">>> Encoders >>>"
        # ">>> Object detection >>>"
        # ">>> Ultrasonic Sensors Detect >>>"
        n129 = call "Elasped Timer.vi"("Time Setting"=5.0, "Action"=Control."Initialize") -> ()  [unwired: 6 in, 4 out]
        n130 = Bundle By Name(cluster=w1364, "Time up flag"=FALSE) -> (w1362:T10)
      }
      frame "START TIMER" {
        # ">>State Logic  >>"
        # ">>> Time cluster >>>"
        # ">>> Yaw >>>"
        # ">>> Stepper position >>>"
        # ">>> Encoders >>>"
        # ">>> Object detection >>>"
        # ">>> Ultrasonic Sensors Detect >>>"
        n131 = call "Elasped Timer.vi"("Action"=Control."Start") -> ("Time Out?!"=w1372:bool)  [unwired: 7 in, 3 out]
        n132 = Bundle By Name(cluster=w1374, "Time up flag"=w1372) -> (w1373:T10)
      }
    }
    "State Logic" <- w222
    n133 = local read "TASK ENABLE"() -> (w216:bool)
    n134 = Not(x=w216) -> (.not. x?=w215:bool)
    n135 = case shown="True" w223 {
      tunnel: w227 -> [w250 w281]
      tunnel: w231 -> [w246 w283]
      tunnel: [w250 w281] -> w236
      tunnel: [w246 w284] -> w235
      tunnel: w232 -> [_ w279]
      tunnel: w234 -> [_ w280]
      tunnel: w229 -> [w249 w286]
      tunnel: [w249 w286] -> w228
      tunnel: "STOP TASK" -> [_ w269]
      tunnel: w222 -> [w248 w285]
      tunnel: [w248 w282] -> w221
      tunnel: w218 -> [w247 w275]
      tunnel: [w247 w275] -> w217
      tunnel: w215 -> [_ w270]
      tunnel: [w245 w267] -> w214
      tunnel: w213 -> [w245 w266]
      tunnel: w209 -> [w244 w263]
      tunnel: [w244 w263] -> w208
      tunnel: w206 -> [w243 w259]
      tunnel: [w243 w259] -> w205
      tunnel: w203 -> [w242 w257]
      tunnel: [w242 w257] -> w202
      tunnel: w200 -> [w241 w255]
      tunnel: [w241 w255] -> w199
      tunnel: w198 -> [w240 w254]
      tunnel: [w240 w253] -> w197
      tunnel: [_ w251] -> w196
      frame False {
        # ">>> yStepper command>>>"
        # ">>> Time cluster >>>"
        # ">>> Yaw >>>"
        # ">>> Stepper position >>>"
        # ">>> Encoders >>>"
        # ">>> Object detection >>>"
        # ">>> Ultrasonic Sensors Detect >>>"
        # ">>> Time cluster >>>"
        # ">>> Yaw >>>"
        # ">>> Stepper position >>>"
        # ">>> Encoders >>>"
        # ">>> Object detection >>>"
        # ">>> Ultrasonic Sensors Detect >>>"
      }
      frame True {
        # ">>State Logic Queue Reference >>"
        # ">>Timeout>>"
        # ">>> yStepper command>>>"
        # ">>> Time cluster >>>"
        # ">>> Object detection >>>"
        # ">>> Yaw >>>"
        # ">>> Ultrasonic Sensors Detect >>>"
        # ">>> Encoders >>>"
        # ">>> Stepper position >>>"
        # ">>State Logic  >>"
        # ">>True Stop Next State >>"
        # ">>Action Queue>>"
        # ">> Manual override >>"
        # ">>> Time cluster >>>"
        # ">>> Yaw >>>"
        # ">>> Stepper position >>>"
        # ">>> Encoders >>>"
        # ">>> Object detection >>>"
        # ">>> Ultrasonic Sensors Detect >>>"
        # ">>Action Queue>>"
        # ">>State Logic Queue Reference >>"
        n136 = Or(x=w269, y=w270) -> (x .or. y?=w268:bool)
        n137 = Unbundle By Name(w257) -> ("Yaw"=w258:dbl, "Compass"=w252:dbl)
        n138 = Unbundle By Name(w255) -> ("Time up flag"=w256:bool)
        "Time up flag" <- w256
        n139 = Unbundle By Name(w259) -> ("y Stepper Position"=w261:u8, "z Stepper Position"=w260:u8)
        n140 = Unbundle By Name(w275) -> ("xDistance"=w272:dbl, "yDistance"=w273:dbl, "wDistance"=w274:dbl)
        n141 = Unbundle By Name(w263) -> ("Recognized Object"=w262:bool, "Object X coordinate"=w265:dbl, "Object Y coordinate"=w264:dbl)
        n142 = Unbundle By Name(w286) -> ("PING_A"=w278:u8, "PING_B"=w277:u8, "PING_C"=w276:u8, "PING_D"=w271:u8)
        n143 = case shown="25" w285 {
          tunnel: [w289 w295 w307 w316 w376 w389 w426 w473 w518 w576 w614 w667 w706 w745 w795 w831 w881 w923] -> w284
          tunnel: w283 -> [w289 w298 w308 w319 w378 w390 w427 w474 w524 w569 w618 w657 w709 w751 w794 w830 w876 w914]
          tunnel: [State_Type_Definitions."Idle" ("Enum") State_Type_Definitions."Idle" ("Enum") w303 w318 State_Type_Definitions."Shutdown" ("Enum") w391 w429 w472 w519 w575 w615 w666 w707 w752 w796 w832 w882 w915] -> w282
          tunnel: w281 -> [_ _ w306 w322 _ w396 w439 w481 w523 w573 w619 w664 w703 w750 w792 w837 w879 w922]
          tunnel: w280 -> [_ _ _ w321 _ w395 w438 w480 w522 w572 w611 w663 w702 w749 w791 w836 w878 w920]
          tunnel: w279 -> [_ _ w305 w317 _ w394 w437 w479 w521 w571 w610 w665 w704 w748 w790 w835 w877 w921]
          tunnel: w268 -> [_ _ _ _ _ w388 w428 w476 w517 w574 w616 w658 w710 w746 w793 w834 w880 w918]
          tunnel: w278 -> [_ _ _ _ _ _ _ _ _ _ _ _ _ _ _ _ _ _]
          tunnel: w277 -> [_ _ _ _ _ _ w435 _ w515 w564 w621 _ _ _ _ _ _ _]
          tunnel: w276 -> [_ _ _ _ _ _ w434 _ w516 w565 w620 _ _ _ _ _ _ _]
          tunnel: w274 -> [_ _ _ _ _ _ _ w478 _ _ _ _ _ _ _ _ _ _]
          tunnel: w273 -> [_ _ _ _ _ w387 _ _ _ _ _ _ _ _ _ _ _ _]
          tunnel: w272 -> [_ _ _ _ _ _ _ _ _ w560 _ _ _ _ _ _ _ _]
          tunnel: w271 -> [_ _ _ _ _ _ _ _ _ _ _ _ _ _ _ _ _ _]
          tunnel: [State_Type_Definitions."Idle" ("Enum") State_Type_Definitions."Idle" ("Enum") State_Type_Definitions."Idle" ("Enum") State_Type_Definitions."Idle" ("Enum") State_Type_Definitions."Shutdown" ("Enum") w384 w425 w469 w510 w559 w613 w668 w708 w744 w797 w833 w883 w916] -> w267
          tunnel: w266 -> [_ _ w303 _ _ _ _ _ _ _ _ _ _ _ _ _ _ _]
          tunnel: w262 -> [_ _ _ _ _ _ _ _ _ _ _ _ _ _ _ _ _ w917]
          tunnel: w265 -> [_ _ _ _ _ _ _ _ _ _ _ _ _ _ _ _ _ _]
          tunnel: w264 -> [_ _ _ _ _ _ _ _ _ _ _ _ _ _ w782 _ _ _]
          tunnel: w261 -> [_ _ _ _ _ _ _ _ _ _ _ _ _ _ w786 _ _ _]
          tunnel: w260 -> [_ _ _ _ _ _ _ _ _ _ _ w661 _ _ _ w838 w875 _]
          tunnel: w258 -> [_ _ _ _ _ _ _ _ _ _ _ _ _ _ _ _ _ _]
          tunnel: w256 -> [_ _ _ _ _ _ _ _ _ _ _ _ w705 w742 _ _ _ _]
          tunnel: w254 -> [w287 w293 w302 w314 w374 w383 w424 w468 w509 w557 w609 w656 w700 w743 w783 w829 w872 w913]
          tunnel: [w287 w292 w302 w314 w374 w383 w424 w468 w509 w557 w609 w656 w700 w743 w788 w829 w872 w913] -> w253
          tunnel: w252 -> [_ _ _ _ _ _ _ _ _ _ _ _ _ _ _ _ _ _]
          tunnel: [_ _ _ TRUE _ _ _ _ _ _ _ _ _ _ _ _ _ _] -> w251
          frame 0 {
            # ">>> yStepper command>>>"
          }
          frame 1 {
            # ">>> yStepper command>>>"
            n144 = for {
              shift-right: [w301] -> w295
              shift-left: w298 -> [w300]
              tunnel: string[] ["INIT", "RESET ARM", "RESET FLAGS", "RESET YAW", "NAVX CALIBRATE"] -> [w299] mode=indexing
              n145 = Enqueue Element(queue=w300, element=w299) -> (queue out=w301:refnum<queue>)  [unwired: 2 in, 2 out]
            }
            n146 = Bundle By Name(cluster=w293, "yStepper desired"=u8 0) -> (w292:T9)
          }
          frame 3 {
            # ">>> yStepper command>>>"
            n147 = Flush Queue(queue=w306, error in (no error)=w305) -> ()  [unwired: 3 out]
            n148 = for {
              shift-right: [w312] -> w307
              shift-left: w308 -> [w311]
              tunnel: string[] ["STOP", "RESET ENCODERS", "RESET YAW", "RESET ARM", "DISPOSE BUFFERS", "CAM CLOSE", ""] -> [w310] mode=indexing
              n149 = Enqueue Element(queue=w311, element=w310) -> (queue out=w312:refnum<queue>)  [unwired: 2 in, 2 out]
            }
          }
          frame 4, Default {
            (unwired) TRUE ("Green LED")
            # ">>> yStepper command>>>"
            n150 = Dequeue Element(queue=w322, timeout in ms (-1)=w321, error in (no error)=w317) -> (element=w320:T8)  [unwired: 3 out]
            n151 = case shown="\"Start Task 6\"" w320 {
              tunnel: [w324 w331 w338 w345 w352 w359 w366 w368] -> w316
              tunnel: w319 -> [w325 w332 w339 w346 w353 w360 w366 w369]
              tunnel: [State_Type_Definitions."Task 1" ("Enum") State_Type_Definitions."Task 2" ("Enum") State_Type_Definitions."Task 3" ("Enum") State_Type_Definitions."Task 4_A" ("Enum") State_Type_Definitions."Task 5_A" ("Enum") State_Type_Definitions."Task 6_A" ("Enum") State_Type_Definitions."Idle" ("Enum") State_Type_Definitions."Shutdown" ("Enum")] -> w318
              frame "Start Task 1" {
                n152 = for {
                  shift-right: [w329] -> w324
                  shift-left: w325 -> [w328]
                  tunnel: string[] ["RESET ENCODERS", "RESET YAW", "FORWARD", "READ ENCODERS"] -> [w327] mode=indexing
                  n153 = Enqueue Element(queue=w328, element=w327) -> (queue out=w329:refnum<queue>)  [unwired: 2 in, 2 out]
                }
              }
              frame "Start Task 2" {
                n154 = for {
                  shift-right: [w336] -> w331
                  shift-left: w332 -> [w335]
                  tunnel: string[] ["RESET ENCODERS", "RESET YAW", "READ ULTRASONIC", "ARDUINO - ULTRASONIC"] -> [w334] mode=indexing
                  n155 = Enqueue Element(queue=w335, element=w334) -> (queue out=w336:refnum<queue>)  [unwired: 2 in, 2 out]
                }
              }
              frame "Start Task 3" {
                n156 = for {
                  shift-right: [w343] -> w338
                  shift-left: w339 -> [w342]
                  tunnel: string[] ["RESET ENCODERS", "READ ENCODERS", "R-ACW"] -> [w341] mode=indexing
                  n157 = Enqueue Element(queue=w342, element=w341) -> (queue out=w343:refnum<queue>)  [unwired: 2 in, 2 out]
                }
              }
              frame "Start Task 4" {
                n158 = for {
                  shift-right: [w350] -> w345
                  shift-left: w346 -> [w349]
                  tunnel: string[] ["STOP", "RESET YAW", "RESET ENCODERS", "ARDUINO - ULTRASONIC", "READ ULTRASONIC", ""] -> [w348] mode=indexing
                  n159 = Enqueue Element(queue=w349, element=w348) -> (queue out=w350:refnum<queue>)  [unwired: 2 in, 2 out]
                }
              }
              frame "Start Task 5" {
                n160 = for {
                  shift-right: [w357] -> w352
                  shift-left: w353 -> [w356]
                  tunnel: string[] ["RESET YAW", "RESET ENCODERS", "READ STEPPER VALUES", "Z STEPPER CAM HEIGHT", "", ""] -> [w355] mode=indexing
                  n161 = Enqueue Element(queue=w356, element=w355) -> (queue out=w357:refnum<queue>)  [unwired: 2 in, 2 out]
                }
              }
              frame "Start Task 6" {
                n162 = for {
                  shift-right: [w364] -> w359
                  shift-left: w360 -> [w363]
                  tunnel: string[] ["OPEN LOG CAM ", "", "", "", "", ""] -> [w362] mode=indexing
                  n163 = Enqueue Element(queue=w363, element=w362) -> (queue out=w364:refnum<queue>)  [unwired: 2 in, 2 out]
                }
              }
              frame "None", Default {
              }
              frame "Exit" {
                n164 = for {
                  shift-right: [w373] -> w368
                  shift-left: w369 -> [w372]
                  tunnel: string[] ["STOP", "RESET ENCODERS", "RESET YAW", "EXIT"] -> [w371] mode=indexing
                  n165 = Enqueue Element(queue=w372, element=w371) -> (queue out=w373:refnum<queue>)  [unwired: 2 in, 2 out]
                }
              }
            }
          }
          frame 5 {
            # ">>> yStepper command>>>"
            n166 = for {
              shift-right: [w382] -> w376
              shift-left: w378 -> [w381]
              tunnel: string[] ["INIT", "RESET ENCODERS", "RESET FLAGS", "EXIT"] -> [w380] mode=indexing
              n167 = Enqueue Element(queue=w381, element=w380) -> (queue out=w382:refnum<queue>)  [unwired: 2 in, 2 out]
            }
          }
          frame 6 {
            # ">>> yStepper command>>>"
            # "Use 250"
            n168 = Dequeue Element(queue=w396, timeout in ms (-1)=w395, error in (no error)=w394) -> (element=w393:T8)  [unwired: 3 out]
            n169 = Greater?(x=w387, y=250.0) -> (0:w385:bool)
            n170 = Or(x=w385, y=w388) -> (x .or. y?=w392:bool)
            n171 = case shown="\"None\", Default" w393 {
              tunnel: w392 -> [w399 _]
              tunnel: [w403 State_Type_Definitions."True Stop" ("Enum")] -> w391
              tunnel: w390 -> [w400 w418]
              tunnel: [w398 w417] -> w389
              tunnel: [State_Type_Definitions."Idle" ("Enum") State_Type_Definitions."Shutdown" ("Enum")] -> w384
              frame "None", Default {
                n172 = case shown="True" w399 {
                  tunnel: w400 -> [w406 w412]
                  tunnel: [w405 w410] -> w398
                  frame False {
                    n173 = for {
                      shift-right: [w408] -> w405
                      shift-left: w406 -> [w409]
                      tunnel: string[] ["READ ENCODERS", "READ YAW", "FORWARD"] ("element") -> [w407] mode=indexing
                      n174 = Enqueue Element(queue=w409, element=w407) -> (queue out=w408:refnum<queue>)  [unwired: 2 in, 2 out]
                    }
                  }
                  frame True {
                    n175 = for {
                      shift-right: [w414] -> w410
                      shift-left: w412 -> [w415]
                      tunnel: string[] ["RESET YAW", "RESET ENCODERS", "STOP", ""] -> [w413] mode=indexing
                      n176 = Enqueue Element(queue=w415, element=w413) -> (queue out=w414:refnum<queue>)  [unwired: 2 in, 2 out]
                    }
                  }
                }
                n177 = Select(t=State_Type_Definitions."True Stop" ("Enum"), s=w399, f=State_Type_Definitions."Task 1" ("Enum")) -> (s? t:f=w403:u16)
              }
              frame "Exit" {
                n178 = for {
                  shift-right: [w422] -> w417
                  shift-left: w418 -> [w423]
                  tunnel: string[] ["STOP", "RESET ENCODERS", "RESET YAW", ""] -> [w421] mode=indexing
                  n179 = Enqueue Element(queue=w423, element=w421) -> (queue out=w422:refnum<queue>)  [unwired: 2 in, 2 out]
                }
              }
            }
          }
          frame 7 {
            w433 = u8 10 ("y")
            # ">>> yStepper command>>>"
            # ">>Object detected>>"
            n180 = Dequeue Element(queue=w439, timeout in ms (-1)=w438, error in (no error)=w437) -> (element=w436:T8)  [unwired: 3 out]
            n181 = Less?(x=w435, y=w433) -> (x < y?=w432:bool)
            n182 = Less?(x=w434, y=w433) -> (x < y?=w431:bool)
            n183 = Or(x=w432, y=w431) -> (x .or. y?=w430:bool)
            "Obstacle detected" <- w430
            n184 = case shown="\"None\", Default" w436 {
              tunnel: w430 -> [w443 _]
              tunnel: [w445 State_Type_Definitions."True Stop" ("Enum")] -> w429
              tunnel: w428 -> [w444 _]
              tunnel: w427 -> [w442 w462]
              tunnel: [w441 w463] -> w426
              tunnel: [State_Type_Definitions."Idle" ("Enum") State_Type_Definitions."Shutdown" ("Enum")] -> w425
              frame "None", Default {
                n185 = case shown="True" w443 {
                  tunnel: w442 -> [w449 w456]
                  tunnel: [w450 w455] -> w441
                  frame False {
                    n186 = for {
                      tunnel: string[] ["READ ULTRASONIC", "STOP"] ("element") -> [w451] mode=indexing
                      shift-right: [w453] -> w450
                      shift-left: w449 -> [w452]
                      n187 = Enqueue Element(queue=w452, element=w451) -> (queue out=w453:refnum<queue>)  [unwired: 2 in, 2 out]
                    }
                  }
                  frame True {
                    n188 = for {
                      shift-right: [w458] -> w455
                      shift-left: w456 -> [w459]
                      tunnel: string[] ["REVERSE", "READ ULTRASONIC", "READ YAW"] -> [w457] mode=indexing
                      n189 = Enqueue Element(queue=w459, element=w457) -> (queue out=w458:refnum<queue>)  [unwired: 2 in, 2 out]
                    }
                  }
                }
                n190 = Select(t=State_Type_Definitions."True Stop" ("Enum"), s=w444, f=State_Type_Definitions."Task 2" ("Enum")) -> (s? t:f=w445:u16)
              }
              frame "Exit" {
                n191 = for {
                  shift-right: [w466] -> w463
                  shift-left: w462 -> [w467]
                  tunnel: string[] ["STOP", "RESET ENCODERS", "RESET YAW", "ARDUINO MODE 0"] -> [w465] mode=indexing
                  n192 = Enqueue Element(queue=w467, element=w465) -> (queue out=w466:refnum<queue>)  [unwired: 2 in, 2 out]
                }
              }
            }
          }
          frame 8 {
            # ">>> yStepper command>>>"
            n193 = Dequeue Element(queue=w481, timeout in ms (-1)=w480, error in (no error)=w479) -> (element=w470:T8)  [unwired: 3 out]
            n194 = Greater?(x=w478, y=100.0) -> (0:w475:bool)
            n195 = Or(x=w475, y=w476) -> (x .or. y?=w471:bool)
            n196 = case shown="\"Exit\"" w470 {
              tunnel: w471 -> [w484 _]
              tunnel: [w488 State_Type_Definitions."True Stop" ("Enum")] -> w472
              tunnel: w474 -> [w485 w504]
              tunnel: [w483 w503] -> w473
              tunnel: [State_Type_Definitions."Idle" ("Enum") State_Type_Definitions."Shutdown" ("Enum")] -> w469
              frame "None", Default {
                n197 = case shown="False" w484 {
                  tunnel: w485 -> [w491 w497]
                  tunnel: [w490 w495] -> w483
                  frame False {
                    n198 = for {
                      shift-right: [w493] -> w490
                      shift-left: w491 -> [w494]
                      tunnel: string[] ["READ ENCODERS", "R-ACW"] ("element") -> [w492] mode=indexing
                      n199 = Enqueue Element(queue=w494, element=w492) -> (queue out=w493:refnum<queue>)  [unwired: 2 in, 2 out]
                    }
                  }
                  frame True {
                    n200 = for {
                      shift-right: [w499] -> w495
                      shift-left: w497 -> [w500]
                      tunnel: string[] ["RESET YAW", "RESET ENCODERS", "STOP", "ARDUINO MODE 0"] -> [w498] mode=indexing
                      n201 = Enqueue Element(queue=w500, element=w498) -> (queue out=w499:refnum<queue>)  [unwired: 2 in, 2 out]
                    }
                  }
                }
                n202 = Select(t=State_Type_Definitions."True Stop" ("Enum"), s=w484, f=State_Type_Definitions."Task 3" ("Enum")) -> (s? t:f=w488:T7)
              }
              frame "Exit" {
                n203 = for {
                  shift-right: [w507] -> w503
                  shift-left: w504 -> [w508]
                  tunnel: string[] ["STOP", "RESET ENCODERS", "RESET YAW", ""] -> [w506] mode=indexing
                  n204 = Enqueue Element(queue=w508, element=w506) -> (queue out=w507:refnum<queue>)  [unwired: 2 in, 2 out]
                }
              }
            }
          }
          frame 9 {
            w514 = u8 20
            # ">>> yStepper command>>>"
            # ">> Outputs true if object detected >>"
            # ">> Manual override >>"
            n205 = Dequeue Element(queue=w523, timeout in ms (-1)=w522, error in (no error)=w521) -> (element=w520:T8)  [unwired: 3 out]
            n206 = Less?(x=w516, y=w514) -> (x < y?=w512:bool)
            n207 = Less?(x=w515, y=w514) -> (x < y?=w513:bool)
            n208 = And(x=w513, y=w512) -> (x .and. y?=w511:bool)
            "Obstacle detected?" <- w511
            n209 = case shown="\"None\", Default" w520 {
              tunnel: [w533 State_Type_Definitions."True Stop" ("Enum")] -> w519
              tunnel: [w531 w552] -> w518
              tunnel: w524 -> [w530 _]
              tunnel: w517 -> [w528 _]
              tunnel: w511 -> [w526 _]
              tunnel: [w525 State_Type_Definitions."Shutdown" ("Enum")] -> w510
              frame "None", Default {
                # ">> WIill proceed to part ii if not manual override >>"
                # ">>If ENABLE or Trigger is set to true>>"
                n210 = Or(x=w526, y=w528) -> (x .or. y?=w527:bool)
                n211 = case shown="True" w527 {
                  tunnel: [w540 w545] -> w531
                  tunnel: w530 -> [w538 w544]
                  frame False {
                    n212 = for {
                      shift-right: [w542] -> w540
                      shift-left: w538 -> [w543]
                      tunnel: string[] ["FORWARD", "READ YAW", "READ ULTRASONIC"] ("element") -> [w541] mode=indexing
                      n213 = Enqueue Element(queue=w543, element=w541) -> (queue out=w542:refnum<queue>)  [unwired: 2 in, 2 out]
                    }
                  }
                  frame True {
                    n214 = for {
                      shift-right: [w548] -> w545
                      shift-left: w544 -> [w549]
                      tunnel: string[] ["STOP", "RESET ENCODERS", "RESET YAW", "ARDUINO - ULTRASONIC"] -> [w547] mode=indexing
                      n215 = Enqueue Element(queue=w549, element=w547) -> (queue out=w548:refnum<queue>)  [unwired: 2 in, 2 out]
                    }
                  }
                }
                n216 = case shown="False" w528 {
                  tunnel: [State_Type_Definitions."True Stop" ("Enum") State_Type_Definitions."True Stop" ("Enum")] -> w529
                  tunnel: [State_Type_Definitions."Task 4_B" ("Enum") State_Type_Definitions."Idle" ("Enum")] -> w525
                  frame False {
                  }
                  frame True {
                  }
                }
                n217 = Select(t=w529, s=w527, f=State_Type_Definitions."Task 4_A" ("Enum")) -> (s? t:f=w533:T7)
              }
              frame "Exit" {
                n218 = for {
                  shift-right: [w555] -> w552
                  shift-left: _ -> [w556]
                  tunnel: string[] ["STOP", "RESET ENCODERS", "RESET YAW", ""] -> [w554] mode=indexing
                  n219 = Enqueue Element(queue=w556, element=w554) -> (queue out=w555:refnum<queue>)  [unwired: 2 in, 2 out]
                }
              }
            }
          }
          frame 10 {
            w568 = 20
            # ">>> yStepper command>>>"
            # ">> Outputs true if 150 mm has been moved >>"
            # ">> Outputs true if sensor not obstructed>>"
            # ">> Manual override >>"
            n220 = Dequeue Element(queue=w573, timeout in ms (-1)=w572, error in (no error)=w571) -> (element=w570:T8)  [unwired: 3 out]
            n221 = Greater?(x=w565, y=w568) -> (0:w566:bool)
            n222 = Greater?(x=w564, y=w568) -> (0:w567:bool)
            n223 = Greater Or Equal?(x=w560, y=80.0) -> (x >= y?=w562:bool)
            n224 = And(x=w567, y=w566) -> (x .and. y?=w561:bool)
            n225 = And(x=w562, y=w561) -> (x .and. y?=w558:bool)
            n226 = case shown="\"None\", Default" w570 {
              tunnel: [w585 State_Type_Definitions."True Stop" ("Enum")] -> w575
              tunnel: [w583 w604] -> w576
              tunnel: w569 -> [w582 _]
              tunnel: w574 -> [w580 _]
              tunnel: w558 -> [w578 _]
              tunnel: [w577 State_Type_Definitions."Shutdown" ("Enum")] -> w559
              frame "None", Default {
                # ">> WIill proceed to part ii if not manual override >>"
                # ">>If ENABLE or Trigger is set to true>>"
                n227 = Or(x=w578, y=w580) -> (x .or. y?=w579:bool)
                n228 = case shown="False" w579 {
                  tunnel: [w592 w597] -> w583
                  tunnel: w582 -> [w590 w596]
                  frame False {
                    n229 = for {
                      shift-right: [w594] -> w592
                      shift-left: w590 -> [w595]
                      tunnel: string[] ["RIGHT", "READ ULTRASONIC", "READ ENCODERS", "READ YAW", "ARDUINO - ULTRASONIC"] ("element") -> [w593] mode=indexing
                      n230 = Enqueue Element(queue=w595, element=w593) -> (queue out=w594:refnum<queue>)  [unwired: 2 in, 2 out]
                    }
                  }
                  frame True {
                    n231 = for {
                      shift-right: [w600] -> w597
                      shift-left: w596 -> [w601]
                      tunnel: string[] ["STOP", "RESET ENCODERS", "RESET YAW", "ARDUINO MODE 0"] -> [w599] mode=indexing
                      n232 = Enqueue Element(queue=w601, element=w599) -> (queue out=w600:refnum<queue>)  [unwired: 2 in, 2 out]
                    }
                  }
                }
                n233 = case shown="True" w580 {
                  tunnel: [State_Type_Definitions."True Stop" ("Enum") State_Type_Definitions."True Stop" ("Enum")] -> w581
                  tunnel: [State_Type_Definitions."Task 4_C" ("Enum") State_Type_Definitions."Idle" ("Enum")] -> w577
                  frame False {
                  }
                  frame True {
                  }
                }
                n234 = Select(t=w581, s=w579, f=State_Type_Definitions."Task 4_B" ("Enum")) -> (s? t:f=w585:T7)
              }
              frame "Exit" {
                n235 = for {
                  shift-right: [w607] -> w604
                  shift-left: _ -> [w608]
                  tunnel: string[] ["STOP", "RESET ENCODERS", "RESET YAW", ""] -> [w606] mode=indexing
                  n236 = Enqueue Element(queue=w608, element=w606) -> (queue out=w607:refnum<queue>)  [unwired: 2 in, 2 out]
                }
              }
            }
          }
          frame 11 {
            w624 = u8 20
            # ">>> yStepper command>>>"
            # ">> Outputs true if object detected >>"
            # ">> Manual override >>"
            n237 = Dequeue Element(queue=w619, timeout in ms (-1)=w611, error in (no error)=w610) -> (element=w612:T8)  [unwired: 3 out]
            n238 = Less?(x=w620, y=w624) -> (x < y?=w622:bool)
            n239 = Less?(x=w621, y=w624) -> (x < y?=w623:bool)
            n240 = And(x=w623, y=w622) -> (x .and. y?=w617:bool)
            n241 = case shown="\"None\", Default" w612 {
              tunnel: [w635 State_Type_Definitions."True Stop" ("Enum")] -> w615
              tunnel: [w633 w651] -> w614
              tunnel: w618 -> [w632 w648]
              tunnel: w616 -> [w629 _]
              tunnel: w617 -> [w630 _]
              tunnel: [w625 State_Type_Definitions."Shutdown" ("Enum")] -> w613
              frame "None", Default {
                # ">> WIill proceed to part ii if not manual override >>"
                # ">>If ENABLE or Trigger is set to true>>"
                n242 = Or(x=w630, y=w629) -> (x .or. y?=w631:bool)
                n243 = case shown="True" w631 {
                  tunnel: [w638 w643] -> w633
                  tunnel: w632 -> [w636 w642]
                  frame False {
                    n244 = for {
                      shift-right: [w640] -> w638
                      shift-left: w636 -> [w641]
                      tunnel: string[] ["FORWARD", "READ ULTRASONIC", "ARDUINO - ULTRASONIC", "READ YAW"] ("element") -> [w639] mode=indexing
                      n245 = Enqueue Element(queue=w641, element=w639) -> (queue out=w640:refnum<queue>)  [unwired: 2 in, 2 out]
                    }
                  }
                  frame True {
                    n246 = for {
                      shift-right: [w646] -> w643
                      shift-left: w642 -> [w647]
                      tunnel: string[] ["STOP", "RESET ENCODERS", "RESET YAW", "ARDUINO - ULTRASONIC"] -> [w645] mode=indexing
                      n247 = Enqueue Element(queue=w647, element=w645) -> (queue out=w646:refnum<queue>)  [unwired: 2 in, 2 out]
                    }
                  }
                }
                n248 = Select(t=State_Type_Definitions."Idle", s=w629, f=State_Type_Definitions."Idle" ("Enum")) -> (s? t:f=w625:T7)
                n249 = Select(t=State_Type_Definitions."True Stop" ("Enum"), s=w631, f=State_Type_Definitions."Task 4_C" ("Enum")) -> (s? t:f=w635:T7)
              }
              frame "Exit" {
                n250 = for {
                  shift-right: [w654] -> w651
                  shift-left: w648 -> [w655]
                  tunnel: string[] ["STOP", "RESET ENCODERS", "RESET YAW", ""] -> [w653] mode=indexing
                  n251 = Enqueue Element(queue=w655, element=w653) -> (queue out=w654:refnum<queue>)  [unwired: 2 in, 2 out]
                }
              }
            }
          }
          frame 13 {
            # ">>> yStepper command>>>"
            # ">> Manual override >>"
            n252 = Dequeue Element(queue=w664, timeout in ms (-1)=w663, error in (no error)=w665) -> (element=w662:T8)  [unwired: 3 out]
            n253 = Equal?(x=w661, y=u8 80) -> (x = y?=w659:bool)
            n254 = case shown="\"None\", Default" w662 {
              tunnel: [w675 State_Type_Definitions."True Stop" ("Enum")] -> w666
              tunnel: [w678 w695] -> w667
              tunnel: [State_Type_Definitions."Idle" ("Enum") State_Type_Definitions."Shutdown" ("Enum")] -> w668
              tunnel: w659 -> [w674 _]
              tunnel: w658 -> [w673 _]
              tunnel: w657 -> [w669 w692]
              frame "None", Default {
                # "Stays in Task 5_A until stepper reaches desired \nheight"
                # "T: Go back to idle, F: Continue with task\""
                # ">> Manual override >>"
                n255 = case shown="True" w674 {
                  tunnel: [w682 w688] -> w678
                  tunnel: w669 -> [w680 w686]
                  frame False {
                    n256 = for {
                      tunnel: string[] ["Z STEPPER CAM HEIGHT", "READ STEPPER VALUES"] ("element") -> [w683] mode=indexing
                      shift-right: [w685] -> w682
                      shift-left: w680 -> [w684]
                      n257 = Enqueue Element(queue=w684, element=w683) -> (queue out=w685:refnum<queue>)  [unwired: 2 in, 2 out]
                    }
                  }
                  frame True {
                    n258 = for {
                      shift-right: [w690] -> w688
                      shift-left: w686 -> [w691]
                      tunnel: string[] ["OPEN LOG CAM", "SET TIMER", ""] -> [w689] mode=indexing
                      n259 = Enqueue Element(queue=w691, element=w689) -> (queue out=w690:refnum<queue>)  [unwired: 2 in, 2 out]
                    }
                  }
                }
                n260 = Or(x=w674, y=w673) -> (x .or. y?=w676:bool)
                n261 = Select(t=State_Type_Definitions."True Stop" ("Enum"), s=w673, f=State_Type_Definitions."Task 5 _B" ("Enum")) -> (s? t:f=w670:u16)
                n262 = Select(t=w670, s=w676, f=State_Type_Definitions."Task 5_A" ("Enum")) -> (s? t:f=w675:u16)
              }
              frame "Exit" {
                n263 = for {
                  shift-right: [w698] -> w695
                  shift-left: w692 -> [w699]
                  tunnel: string[] ["STOP", "RESET ENCODERS", "RESET YAW", "ARDUINO MODE 0"] -> [w697] mode=indexing
                  n264 = Enqueue Element(queue=w699, element=w697) -> (queue out=w698:refnum<queue>)  [unwired: 2 in, 2 out]
                }
              }
            }
          }
          frame 14 {
            # ">>> yStepper command>>>"
            n265 = Dequeue Element(queue=w703, timeout in ms (-1)=w702, error in (no error)=w704) -> (element=w701:T8)  [unwired: 3 out]
            n266 = case shown="\"None\", Default" w701 {
              tunnel: [w717 State_Type_Definitions."True Stop" ("Enum")] -> w707
              tunnel: [w720 w737] -> w706
              tunnel: [State_Type_Definitions."Idle" ("Enum") State_Type_Definitions."Shutdown" ("Enum")] -> w708
              tunnel: w705 -> [w716 _]
              tunnel: w710 -> [w715 _]
              tunnel: w709 -> [w711 w734]
              frame "None", Default {
                # "Stays in Task 5_B to capture image over 5 seconds"
                # "T: Go back to idle, F: Continue with task\""
                # ">> Manual override >>"
                n267 = case shown="False" w716 {
                  tunnel: [w724 w730] -> w720
                  tunnel: w711 -> [w722 w728]
                  frame False {
                    n268 = for {
                      tunnel: string[] ["CAM ACQ", "START TIMER", ""] ("element") -> [w725] mode=indexing
                      shift-right: [w727] -> w724
                      shift-left: w722 -> [w726]
                      n269 = Enqueue Element(queue=w726, element=w725) -> (queue out=w727:refnum<queue>)  [unwired: 2 in, 2 out]
                    }
                  }
                  frame True {
                    n270 = for {
                      shift-right: [w732] -> w730
                      shift-left: w728 -> [w733]
                      tunnel: string[] ["CAM CLOSE", "SET TIMER", "", ""] -> [w731] mode=indexing
                      n271 = Enqueue Element(queue=w733, element=w731) -> (queue out=w732:refnum<queue>)  [unwired: 2 in, 2 out]
                    }
                  }
                }
                n272 = Or(x=w716, y=w715) -> (x .or. y?=w718:bool)
                n273 = Select(t=State_Type_Definitions."True Stop" ("Enum"), s=w715, f=State_Type_Definitions."Task 5_C" ("Enum")) -> (s? t:f=w712:u16)
                n274 = Select(t=w712, s=w718, f=State_Type_Definitions."Task 5 _B" ("Enum")) -> (s? t:f=w717:u16)
              }
              frame "Exit" {
                n275 = for {
                  shift-right: [w740] -> w737
                  shift-left: w734 -> [w741]
                  tunnel: string[] ["STOP", "RESET ENCODERS", "RESET YAW", "ARDUINO MODE 0"] -> [w739] mode=indexing
                  n276 = Enqueue Element(queue=w741, element=w739) -> (queue out=w740:refnum<queue>)  [unwired: 2 in, 2 out]
                }
              }
            }
          }
          frame 15 {
            # ">>> yStepper command>>>"
            # ">> Manual override >>"
            n277 = Dequeue Element(queue=w750, timeout in ms (-1)=w749, error in (no error)=w748) -> (element=w747:T8)  [unwired: 3 out]
            n278 = case shown="\"None\", Default" w747 {
              tunnel: [w757 State_Type_Definitions."True Stop" ("Enum")] -> w752
              tunnel: [w760 w777] -> w745
              tunnel: [State_Type_Definitions."Idle" ("Enum") State_Type_Definitions."Shutdown" ("Enum")] -> w744
              tunnel: w746 -> [w754 _]
              tunnel: w751 -> [w756 w774]
              tunnel: w742 -> [w753 _]
              frame "None", Default {
                # ">> Is object in range? >>"
                # "Determines if object is in range to pick up"
                # ">> Manual override >>"
                n279 = case shown="True" w753 {
                  tunnel: [w764 w770] -> w760
                  tunnel: w756 -> [w762 w768]
                  frame False {
                    n280 = for {
                      tunnel: string[] ["PROCESS IMAGE", "START TIMER"] ("element") -> [w765] mode=indexing
                      shift-right: [w767] -> w764
                      shift-left: w762 -> [w766]
                      n281 = Enqueue Element(queue=w766, element=w765) -> (queue out=w767:refnum<queue>)  [unwired: 2 in, 2 out]
                    }
                  }
                  frame True {
                    n282 = for {
                      shift-right: [w772] -> w770
                      shift-left: w768 -> [w773]
                      tunnel: string[] ["CAM CLOSE", ""] -> [w771] mode=indexing
                      n283 = Enqueue Element(queue=w773, element=w771) -> (queue out=w772:refnum<queue>)  [unwired: 2 in, 2 out]
                    }
                  }
                }
                n284 = Or(x=w753, y=w754) -> (x .or. y?=w758:bool)
                n285 = Select(t=State_Type_Definitions."Task 5_D" ("Enum"), s=w758, f=State_Type_Definitions."Task 5_C_Error" ("Enum")) -> (s? t:f=w757:u16)
              }
              frame "Exit" {
                n286 = for {
                  shift-right: [w780] -> w777
                  shift-left: w774 -> [w781]
                  tunnel: string[] ["STOP", "RESET ENCODERS", "RESET YAW", "ARDUINO MODE 0"] -> [w779] mode=indexing
                  n287 = Enqueue Element(queue=w781, element=w779) -> (queue out=w780:refnum<queue>)  [unwired: 2 in, 2 out]
                }
              }
            }
          }
          frame 15 {
            # ">>> yStepper command>>>"
            # ">> Checks if yStepper has reached target>>"
            n288 = Dequeue Element(queue=w792, timeout in ms (-1)=w791, error in (no error)=w790) -> (element=w789:T8)  [unwired: 3 out]
            n289 = formula code="if (pos >= 160 && pos <= 180)\ny = 25;\nif (pos >= 181 &&pos <= 200) \ny = 20;\n\nelse if (pos >= 201 && pos <= 240)\ny = 15;\n\nelse if (pos >= 241 && pos <= 280)\ny = 10;\n\nelse if (pos >= 281 && pos <= 300)\ny = 5;\n\nelse if (pos > 300)\ny = 0;\n\nelse if (pos == 0 || pos < 100)\ny = 0;"("pos"=w782) -> ("y"=w787:dbl)
            n290 = To Unsigned Byte Integer(number=w787) -> (unsigned 8bit integer=w785:u8)
            n291 = Equal?(x=w786, y=w785) -> (x = y?=w784:bool)
            n292 = case shown="\"None\", Default" w789 {
              tunnel: [w804 State_Type_Definitions."True Stop" ("Enum")] -> w796
              tunnel: [w807 w824] -> w795
              tunnel: [State_Type_Definitions."Idle" ("Enum") State_Type_Definitions."Shutdown" ("Enum")] -> w797
              tunnel: w793 -> [w803 _]
              tunnel: w794 -> [w799 w821]
              tunnel: w784 -> [w798 _]
              frame "None", Default {
                # ">> T: Breaks out of state loop; F: Stays in loop>>"
                # ">> Manual override >>"
                # ">> Checks if yStepper has reached target>>"
                # "Stays in Task 5_C until time is up and object is detected"
                # "T: Go back to idle, F: Continue with task\""
                # ">> Manual override >>"
                n293 = case shown="True" w798 {
                  tunnel: [w811 w817] -> w807
                  tunnel: w799 -> [w809 w815]
                  frame False {
                    n294 = for {
                      tunnel: string[] ["Y STEPPER CONTROL", "READ STEPPER VALUES", ""] ("element") -> [w812] mode=indexing
                      shift-right: [w814] -> w811
                      shift-left: w809 -> [w813]
                      n295 = Enqueue Element(queue=w813, element=w812) -> (queue out=w814:refnum<queue>)  [unwired: 2 in, 2 out]
                    }
                  }
                  frame True {
                    n296 = for {
                      shift-right: [w819] -> w817
                      shift-left: w815 -> [w820]
                      tunnel: string[] ["OPEN LOG CAM", "CAM ACQ", "SET TIMER"] -> [w818] mode=indexing
                      n297 = Enqueue Element(queue=w820, element=w818) -> (queue out=w819:refnum<queue>)  [unwired: 2 in, 2 out]
                    }
                  }
                }
                n298 = Or(x=w798, y=w803) -> (x .or. y?=w805:bool)
                n299 = Select(t=State_Type_Definitions."True Stop" ("Enum"), s=w803, f=State_Type_Definitions."Task 5_D" ("Enum")) -> (s? t:f=w800:u16)
                n300 = Select(t=w800, s=w805, f=State_Type_Definitions."Task 5_C_Error" ("Enum")) -> (s? t:f=w804:u16)
              }
              frame "Exit" {
                n301 = for {
                  shift-right: [w827] -> w824
                  shift-left: w821 -> [w828]
                  tunnel: string[] ["STOP", "RESET ENCODERS", "RESET YAW", "ARDUINO MODE 0"] -> [w826] mode=indexing
                  n302 = Enqueue Element(queue=w828, element=w826) -> (queue out=w827:refnum<queue>)  [unwired: 2 in, 2 out]
                }
              }
            }
            n303 = Bundle By Name(cluster=w783, "yStepper desired"=w785) -> (w788:T9)
          }
          frame 16 {
            # ">>> yStepper command>>>"
            # ">> Manual override >>"
            n304 = Dequeue Element(queue=w837, timeout in ms (-1)=w836, error in (no error)=w835) -> (element=w841:T8)  [unwired: 3 out]
            n305 = Equal?(x=w838, y=u8 1) -> (x = y?=w839:bool)
            n306 = case shown="\"None\", Default" w841 {
              tunnel: [w848 State_Type_Definitions."True Stop" ("Enum")] -> w832
              tunnel: [w851 w867] -> w831
              tunnel: [State_Type_Definitions."Idle" ("Enum") State_Type_Definitions."Shutdown" ("Enum")] -> w833
              tunnel: w839 -> [w847 _]
              tunnel: w834 -> [w842 _]
              tunnel: w830 -> [w843 _]
              frame "None", Default {
                # ">> Break out of loop >>"
                # ">> Height reached >>"
                # ">> Manual override >>"
                # "Stays in Task 5_D until stepper reaches desired \nheight"
                # "T: Go back to idle, F: Continue with task\""
                # ">> Manual override >>"
                n307 = case shown="True" w847 {
                  tunnel: [w855 w861] -> w851
                  tunnel: w843 -> [w853 w859]
                  frame False {
                    n308 = for {
                      tunnel: string[] ["Z STEPPER GRAB HEIGHT", "READ STEPPER VALUES"] ("element") -> [w856] mode=indexing
                      shift-right: [w858] -> w855
                      shift-left: w853 -> [w857]
                      n309 = Enqueue Element(queue=w857, element=w856) -> (queue out=w858:refnum<queue>)  [unwired: 2 in, 2 out]
                    }
                  }
                  frame True {
                    n310 = for {
                      shift-right: [w863] -> w861
                      shift-left: w859 -> [w864]
                      tunnel: string[] ["READ STEPPER VALUES", "", ""] -> [w862] mode=indexing
                      n311 = Enqueue Element(queue=w864, element=w862) -> (queue out=w863:refnum<queue>)  [unwired: 2 in, 2 out]
                    }
                  }
                }
                n312 = Or(x=w847, y=w842) -> (x .or. y?=w849:bool)
                n313 = Select(t=State_Type_Definitions."True Stop" ("Enum"), s=w842, f=State_Type_Definitions."Task 5_D" ("Enum")) -> (s? t:f=w844:u16)
                n314 = Select(t=w844, s=w849, f=State_Type_Definitions."Task 5_D" ("Enum")) -> (s? t:f=w848:u16)
              }
              frame "Exit" {
                n315 = for {
                  shift-right: [w870] -> w867
                  shift-left: _ -> [w871]
                  tunnel: string[] ["STOP", "RESET ENCODERS", "RESET YAW", "ARDUINO MODE 0"] -> [w869] mode=indexing
                  n316 = Enqueue Element(queue=w871, element=w869) -> (queue out=w870:refnum<queue>)  [unwired: 2 in, 2 out]
                }
              }
            }
          }
          frame 25 {
            # ">>> yStepper command>>>"
            n317 = Dequeue Element(queue=w879, timeout in ms (-1)=w878, error in (no error)=w877) -> (element=w884:T8)  [unwired: 3 out]
            n318 = Equal?(x=w875, y=u8 80) -> (x = y?=w874:bool)
            n319 = case shown="\"None\", Default" w884 {
              tunnel: [w891 State_Type_Definitions."True Stop" ("Enum")] -> w882
              tunnel: [w890 w908] -> w881
              tunnel: [State_Type_Definitions."Idle" ("Enum") State_Type_Definitions."Shutdown" ("Enum")] -> w883
              tunnel: w880 -> [w886 _]
              tunnel: w876 -> [w888 _]
              tunnel: w874 -> [w885 _]
              frame "None", Default {
                n320 = case shown="True" w885 {
                  tunnel: [w896 w902] -> w890
                  tunnel: w888 -> [w894 w900]
                  frame False {
                    n321 = for {
                      tunnel: string[] ["Z STEPPER CAM HEIGHT", "READ STEPPER VALUES"] ("element") -> [w897] mode=indexing
                      shift-right: [w899] -> w896
                      shift-left: w894 -> [w898]
                      n322 = Enqueue Element(queue=w898, element=w897) -> (queue out=w899:refnum<queue>)  [unwired: 2 in, 2 out]
                    }
                  }
                  frame True {
                    n323 = for {
                      shift-right: [w904] -> w902
                      shift-left: w900 -> [w905]
                      tunnel: string[] ["CAM ACQ", "OPEN LOG CAM"] -> [w903] mode=indexing
                      n324 = Enqueue Element(queue=w905, element=w903) -> (queue out=w904:refnum<queue>)  [unwired: 2 in, 2 out]
                    }
                  }
                }
                n325 = Or(x=w885, y=w886) -> (x .or. y?=w887:bool)
                n326 = Select(t=State_Type_Definitions."Task 6_B" ("Enum"), s=w887, f=State_Type_Definitions."Task 6_A" ("Enum")) -> (s? t:f=w891:T7)
              }
              frame "Exit" {
                n327 = for {
                  shift-right: [w911] -> w908
                  shift-left: _ -> [w912]
                  tunnel: string[] ["STOP", "RESET ENCODERS", "RESET YAW", "ARDUINO MODE 0"] -> [w910] mode=indexing
                  n328 = Enqueue Element(queue=w912, element=w910) -> (queue out=w911:refnum<queue>)  [unwired: 2 in, 2 out]
                }
              }
            }
          }
          frame 26 {
            # ">>> yStepper command>>>"
            n329 = Dequeue Element(queue=w922, timeout in ms (-1)=w920, error in (no error)=w921) -> (element=w919:T8)  [unwired: 3 out]
            n330 = case shown="\"None\", Default" w919 {
              tunnel: [w929 State_Type_Definitions."True Stop" ("Enum")] -> w915
              tunnel: [w928 w947] -> w923
              tunnel: [State_Type_Definitions."Idle" ("Enum") State_Type_Definitions."Shutdown" ("Enum")] -> w916
              tunnel: w918 -> [w924 _]
              tunnel: w917 -> [w926 _]
              tunnel: w914 -> [w925 w944]
              frame "None", Default {
                # ">> Manual override >>"
                n331 = case shown="True" w926 {
                  tunnel: [w934 w940] -> w928
                  tunnel: w925 -> [w933 w938]
                  frame False {
                    n332 = for {
                      shift-right: [w937] -> w934
                      shift-left: w933 -> [w936]
                      tunnel: string[] ["CAM ACQ", "PROCESS IMAGE", "OPEN CLAW"] -> [w935] mode=indexing
                      n333 = Enqueue Element(queue=w936, element=w935) -> (queue out=w937:refnum<queue>)  [unwired: 2 in, 2 out]
                    }
                  }
                  frame True {
                    n334 = for {
                      shift-right: [w942] -> w940
                      shift-left: w938 -> [w943]
                      tunnel: string[] ["CAM ACQ", "PROCESS IMAGE", "CLOSE CLAW"] -> [w941] mode=indexing
                      n335 = Enqueue Element(queue=w943, element=w941) -> (queue out=w942:refnum<queue>)  [unwired: 2 in, 2 out]
                    }
                  }
                }
                n336 = Select(t=State_Type_Definitions."True Stop" ("Enum"), s=w924, f=State_Type_Definitions."Task 6_B" ("Enum")) -> (s? t:f=w929:T7)
              }
              frame "Exit" {
                # ">> State after true stop >>"
                # ">> Goes to true stop >>"
                n337 = for {
                  shift-right: [w950] -> w947
                  shift-left: w944 -> [w951]
                  tunnel: string[] ["STOP", "RESET ENCODERS", "RESET YAW", ""] -> [w949] mode=indexing
                  n338 = Enqueue Element(queue=w951, element=w949) -> (queue out=w950:refnum<queue>)  [unwired: 2 in, 2 out]
                }
              }
            }
          }
        }
        "Cluster" <- w263
      }
    }
    n339 = local write "Green LED"(w196) -> ()
  }
  n340 = call <vilib>:"DIO Close.vi"("error in (no error)"=w24, "DIO Info In"=w27) -> ()  [unwired: 9 in, 1 out]
  n341 = call <vilib>:"DIO Close.vi"("error in (no error)"=w34, "DIO Info In"=w36) -> ()  [unwired: 9 in, 1 out]
  n342 = call <vilib>:"NavX Close.vi"("error in (no error)"=w5, "NavX Info In"=w4) -> ()  [unwired: 9 in, 1 out]
  n343 = call <vilib>:"DIO Close.vi"("error in (no error)"=w29, "DIO Info In"=w31) -> ()  [unwired: 9 in, 1 out]
  n344 = call <vilib>:"DIO Close.vi"("error in (no error)"=w12, "DIO Info In"=w13) -> ()  [unwired: 9 in, 1 out]
  n345 = call <vilib>:"DIO Close.vi"("error in (no error)"=w7, "DIO Info In"=w8) -> ()  [unwired: 9 in, 1 out]
  n346 = while {
    stop <- w1383 stop-if-true
    n347 = call <vilib>:"RT Get CPU Loads.vi"() -> ("CPU loads"=→"CPU loads":T6[])  [unwired: 10 in, 1 out]
    n348 = Wait (ms)(milliseconds to wait=u32 100) -> ()  [unwired: 1 out]
    n349 = call "FGV Bool.vi"("Init/Read/Write State"=States_for_Action_Engine."Read") -> ("Output node"=w1383:bool)  [unwired: 2 in, 1 out]
  }
  n350 = Merge Errors "Merge Errors"(w64, w63) -> (w46:errorcluster)
  n351 = Merge Errors(w50, w46) -> (w45:errorcluster)
  n352 = Destroy User Event(user event=w67, error in=w45) -> ()  [unwired: 1 out]
  n353 = Destroy User Event(user event=w68, error in=w45) -> ()  [unwired: 1 out]
  n354 = Unregister For Events(event registration refnum=w59, error in=w45) -> ()  [unwired: 1 out]
  n355 = Release Queue(queue=w41, error in (no error)=w45) -> (error out=w23:errorcluster)  [unwired: 1 in, 2 out]
  n356 = Release Queue(queue=w58, error in (no error)=w45) -> ()  [unwired: 1 in, 3 out]
  n357 = call <vilib>:"Simple Error Handler.vi"("error in (no error)"=w23) -> ("error out"=w22:errorcluster)  [unwired: 4 in, 4 out]
  n358 = call <vilib>:"Reset myRIO.vi"("error in (no error)"=w22) -> ("error out"=→"error out":errorcluster)  [unwired: 10 in]
